vi "Find Average Center.vi"(5 "Position":i32, 6 "Database Entry in":refnum<class "Database Entry.lvclass">, 7 "Tray Number":i32, 8 "Assembly Type":string, 9 "XYZTheta":dbl[](array[numeric]), 10 "Sensor Thickness":dbl, 11 "Gantry In":refnum<k24>) -> (1 "XYZTheta":dbl[](array[numeric]) format="%.6g", 3 "Gantry Out":refnum<k24>, 4 "Database Entry out":refnum<class "Database Entry.lvclass">)   [LabVIEW 2021, in "Component Tray.lvclass"]
uses:
  Component Tray.lvclass
  Find Component.ctl
  Controller/Camera/Machine Vision.ctl
  C:/Program Files (x86)/Aerotech/A3200/LabVIEW/2010/Bin/Aerotech.A3200.dll
  Program Files (x86)/Aerotech/A3200/LabVIEW/2010/Bin/Aerotech.A3200.dll
  Controller/Camera/Camera settings.ctl
  <vilib>/vision/Pattern Matching.llb/IMAQ Pattern Match Advanced Options.ctl
  Assembly/Database Entry/Database Entry.lvclass
  Controller/Camera/Edmund Optics/Edmund Optics.lvclass
  C:/Users/HEP/Documents/GitHub/Gantry/UCSB-Gantry-HEP-main/Classes/Controller/Camera/Camera.lvclass
  <vilib>/picture/picture.llb/Draw 4-Bit Pixmap.vi
  Controller/Camera/Camera.lvclass
  Controller/Motion/A3200/A3200.lvclass
  Controller/Motion/Motion.lvclass
  <vilib>/vision/NI_Vision_Development_Module.lvlib
  <vilib>/vision/Image Controls.llb/IMAQ Image.ctl
  <vilib>/vision/driver/NI_Vision_Acquisition_Software.lvlib
panel:
  out "Sensor ID match DB?":bool
  in  "Algorithm":i32(ring)=2 items=["All", "Low Discrepancy Sampling", "Grayscale Value Pyramid", "Gradients Pyramid"]
  in  "Parameters":T1={"Number of Matches Requested"=1, "Minimum Match Score"=800.0, "Angle Ranges"=[]}
  in  "ROI Descriptor":T2 {"Contours"."Type" items=["No Selection", "Point", "Line", "Rectangle", "Oval", "Polygon", "Freehand Region", "Annulus", "Unused2", "Unused3", "Broken Line", "Freehand Line", "Rotated Rectangle"]}
  in  "Advanced Options":cluster{"Item":T3, "Value":dbl}[](array[cluster]) {"Item" items=["LD Sampling - Minimum Constrast"=0, "LD Sampling - Enable Subpixel Accuracy"=1, "LD Sampling - Search Strategy"=2, "LD Sampling - Subpixel Iterations"=3, "LD Sampling - Subpixel Tolerance"=4, "LD Sampling - Initial Match List Length"=5, "LD Sampling - Match List Reduction Factor"=6, "LD Sampling - Initial Step Size"=7, "LD Sampling - Intermediate Angular Accuracy"=8, "-"=9, "Pyramid - Max Pyramid Level"=100, "Pyramid - Minimum Contrast"=102, "Pyramid - Enable Subpixel Accuracy"=103, "Pyramid - Subpixel Iterations"=104, "Pyramid - Subpixel Tolerance"=105, "Pyramid - Initial Match List Length"=106, "Pyramid - Match List Reduction Factor"=107, "Pyramid - Intermediate Angular Accuracy"=108, "Pyramid - Process Border Matches"=109, "Pyramid - Min Match Separation Distance"=111, "Pyramid - Min Match Separation Angle"=112, "Pyramid - Max Match Overlap"=113, "Pyramid - Max Cache in MB"=114, "Pyramid - Clear Cache"=115, "Pyramid - Enable Accurate Score Computation"=116, "Pyramid - Interpolation Method For Score Computation"=117, "Pyramid - Enable Target To Template Score"=118, "-"=119, "Enable Defect Map"=200]}
  out "Sensor ID digits":i32[](array[numeric])
  out "Checking Sensor ID":bool
  out "All Matches XY":sgl[][](array[numeric])
  out "Match found?":bool
  in  "Focus":bool
  out "Gantry":dbl[](array[numeric]) format="%.6g"
  out "Sum":dbl[](array[numeric]) format="%.6g"
  in  "Machine Vision":T4
  out "Radius (Real-World)":dbl
  out "Standard Variation":sgl
  out "Maximal Value":sgl
  out "Average Strength":dbl
  out "Instructions":string
  out "Camera":dbl[](array[numeric])
  out "Image":T5(plugin-control)
  in  "Enter Manual Mode":bool
  out "Manual Mode On":bool
  in  "Auto Submit":bool
  out "Tray and Position":string
  out "Sensor ID":picture[](array[picture])
  out "Sensor ID":string
  out "predicted fiducials":dbl[][](array[numeric])
  out "Current Z High Speed":dbl
  out "Current XY High Speed":dbl
  out "current Z low speed":dbl
  out "current XY speed":dbl
  in  "Z high":dbl=12.5
  in  "XY high":dbl=50.0
  in  "Z low":dbl=0.05
  in  "XY low":dbl=0.1
  in  "Predict fiducials":bool
  out "Low Speed":bool
  out "X":bool
  out "Y":bool
  out "Z":bool
  out "High Speed":bool
  in  "Go to CH191/FD5":bool
  in  "Go to CH197/FD4":bool
  out "Program Done?":bool
  out "Sensor ID Location":dbl[](array[numeric])
  in  "Go to Sensor ID":bool
  out "CH1 XYZ":dbl[](array[numeric])
  out "CH1 correct?":bool
  in  "Go to CH1":bool
  out "All fiducials recorded":bool
  in  "Override camera presets":bool
  in  "Camera settings":T6={"Gamma"=1.6, "Gain"=0, "Sharpness"=0, "Contrast"=0.0, "Exposure"=0.0078125} {"Exposure" min=0.000244140625 max=0.5 scale=0.0002..0.5; "Contrast" min=0.0 max=1.0 scale=0.001..1.0; "Sharpness" min=0 max=2 step=1 scale=0.0..2.0; "Gain" min=0 max=100 step=1 scale=0.1..100.0; "Gamma" min=0.01 max=10.0 scale=0.01..10.0}
  out "CH197/FD4 XYZ":dbl[](array[numeric]) format="%.6g"
  out "CH8/FD2 XYZ":dbl[](array[numeric]) format="%.6g"
  out "CH191/FD5 XYZ":dbl[](array[numeric]) format="%.6g"
  out "CH1/FD1 XYZ":dbl[](array[numeric]) format="%.6g"
  in  "Record CH8/FD2":bool
  in  "Record CH197/FD4":bool
  in  "Record CH191/FD5":bool
  in  "Record CH1/FD1":bool
  in  "Go to CH8/FD2":bool
  in  "Go to CH1/FD1":bool
  in  "Joystick":bool
  in  "Go to Center":bool
  in  "Component":T7
  in  "Stop Program":bool
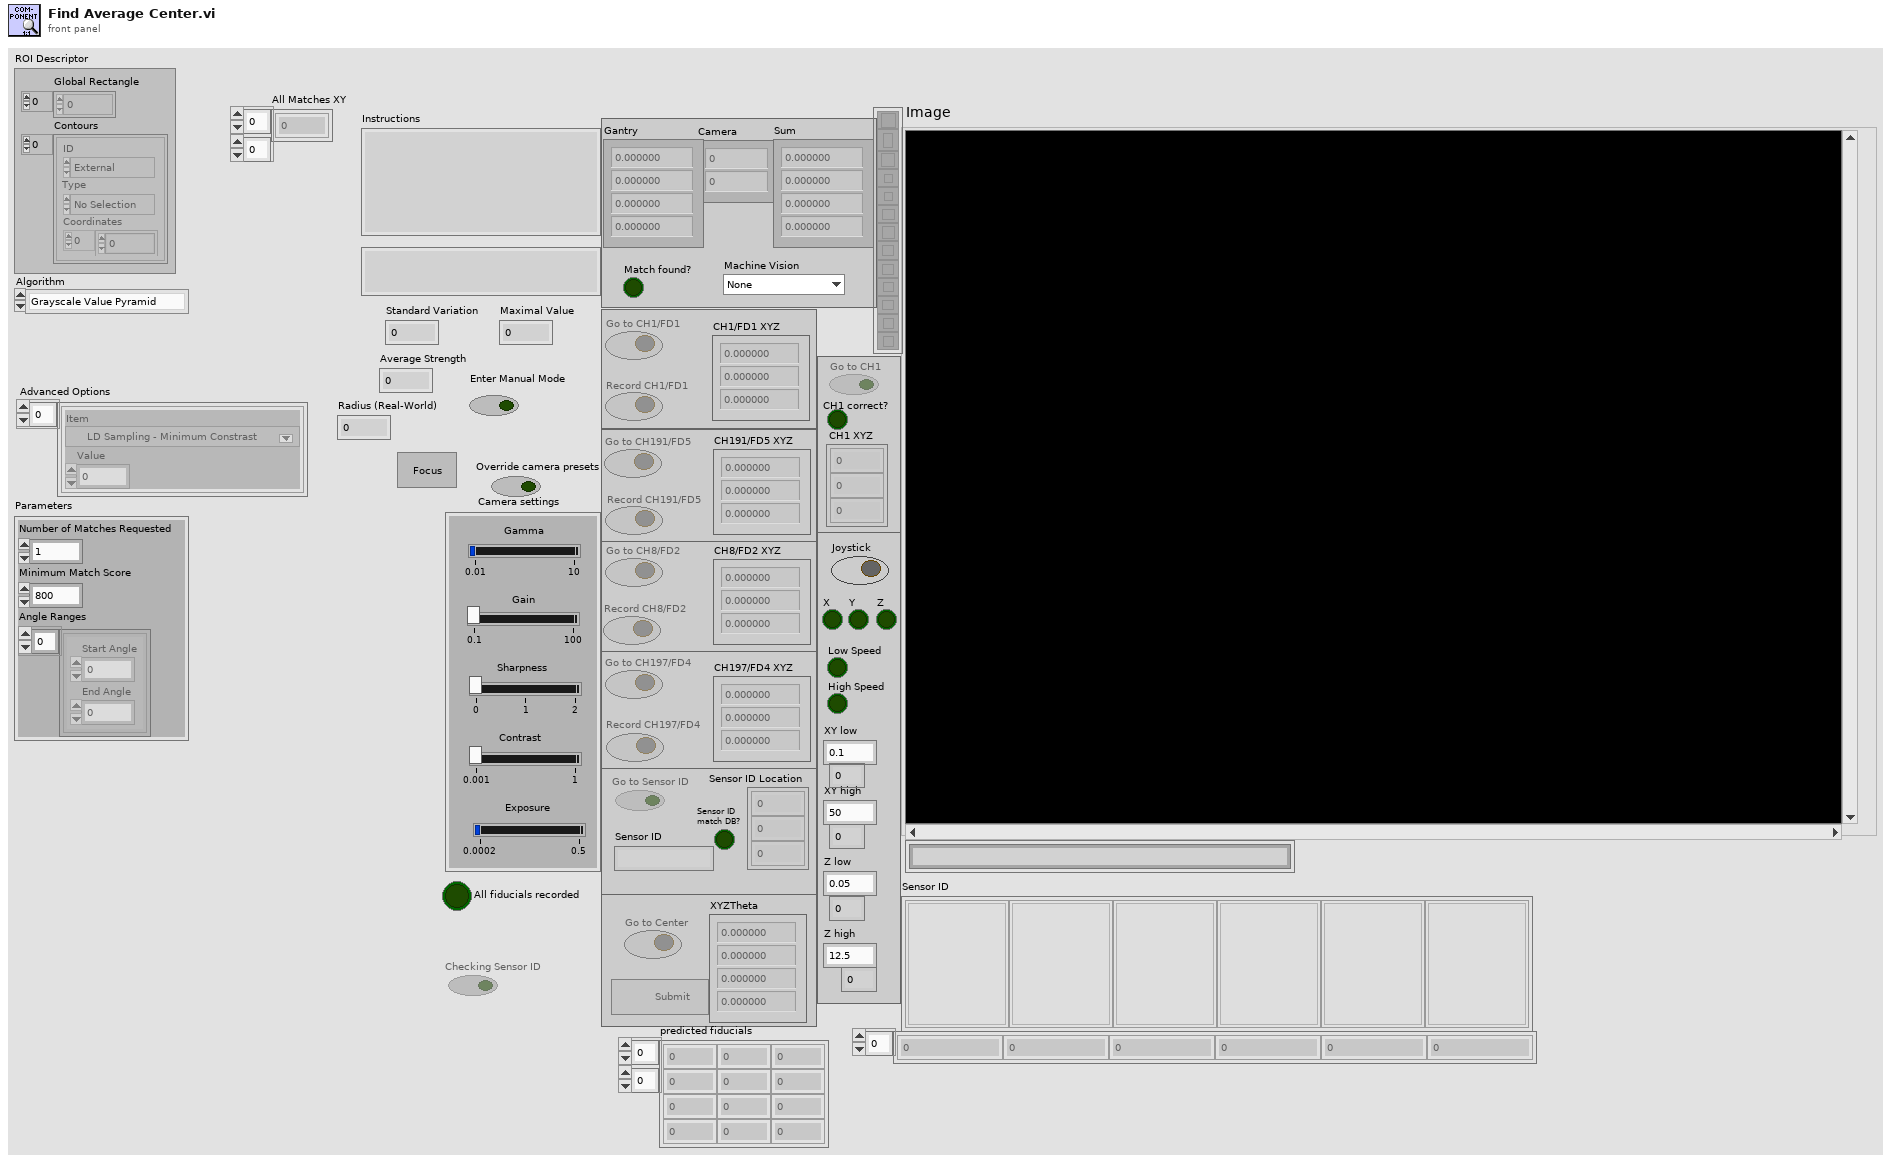
[diagram p1: front panel]
types:
  T1 = cluster{"Number of Matches Requested":i32, "Minimum Match Score":sgl, "Angle Ranges":cluster{"Start Angle":sgl, "End Angle":sgl}[]}
  T2 = typedef "ROI Descriptor" = cluster{"Global Rectangle":i32[], "Contours":cluster{"ID":enum32{"External", "Internal"}, "Type":u32, "Coordinates":i32[]}[]}
  T3 = typedef "IMAQ Pattern Match Advanced Options.ctl" = u16
  T4 = typedef "Camera.lvclass/Machine Vision.ctl" = enum16{"None", "Assembly Tray Circle", "Assembly Tray Fiducial", "Partial Hexaboard", "sensor edge init", "HB edge init", "sensor edge pos1", "sensor edge pos2", "HB edge pos1", "HB edge pos2", "Sensor CH1-2", "HB CH1", "HB CH2", "V3 Sensor Circle", "Hexaboard Circle", "sensor CH1 check", "HB CH1 check ", "sensor ID"}
  T5 = typedef "IMAQ Image.ctl" = refnum<image>
  T6 = typedef "Camera.lvclass/Camera settings.ctl" = cluster{"Gamma":dbl, "Gain":i64, "Sharpness":i64, "Contrast":dbl, "Exposure":dbl}
  T7 = typedef "Component Tray.lvclass/Find Component.ctl" = cluster{"New Fiducials":dbl[], "Past Fiducials":dbl[][], "XYZTheta":dbl[], "Fiducials Path":path, "Position":i32, "CH1 Location":dbl[], "Sensor ID Location":dbl[], "initial rotation":dbl[], "CH2 location":dbl[], "max std variation":dbl, "max strength":dbl, "CH2 pattern matching":T4, "Fiducial Circle":T4, "Get Edge":T4, "Pos multiplier":dbl, "time to wait":u32, "fiducial to edge":dbl, "Protomodule?":bool, "Assembly Type":string, "CH1 to CH2":dbl, "Tray Number":string, "fiducial radius":dbl, "4 fiducials?":bool, "CH1 check":T4, "Edge Scan":T4, "CH1 pattern matching":T4, "Sensor Thickness":dbl, "Previous Avgs":dbl[][], "avg value count":dbl[]}
  T8 = enum8{"Enabled", "Disabled", "Disabled and Grayed Out"}
  T9 = enum16{"None", "Assembly Tray Circle", "Assembly Tray Fiducial", "Partial Hexaboard", "sensor edge init", "HB edge init", "sensor edge pos1", "sensor edge pos2", "HB edge pos1", "HB edge pos2", "Sensor CH1-2", "HB CH1", "HB CH2", "V3 Sensor Circle", "Hexaboard Circle", "sensor CH1 check", "HB CH1 check "}
  T10 = cluster{"Average Strength":dbl, "Radius (Real-World)":dbl, "Match found?":bool, "initial angle":sgl, "Global Report":cluster{"Mean Value":sgl, "Standard Variation":sgl, "Minimal Value":sgl, "Maximal Value":sgl, "Area (calibrated)":sgl, "Area (pixels)":u32, "%":sgl, "Calibration Valid":bool}}
  T11 = typedef "IMAQ GM Match Report.ctl" = cluster{"Position":cluster{"x":sgl, "y":sgl}, "Angle":sgl, "Scale":sgl, "Score":sgl, "Bounding Box":cluster{"x":sgl, "y":sgl}[], "Contrast Reversed":bool, "Occlusion %":sgl, "Template Target Curve Score":sgl, "Target Template Curve Score":sgl, "Correlation Score":sgl}
  T12 = cluster{"Mean Value":sgl, "Standard Variation":sgl, "Minimal Value":sgl, "Maximal Value":sgl, "Area (calibrated)":sgl, "Area (pixels)":u32, "%":sgl, "Calibration Valid":bool}
  T13 = cluster{"left":i16, "top":i16, "right":i16, "bottom":i16}
  T14 = cluster{"Algorithm":i32, "Number of Matches Requested":i32, "Minimum Match Score":sgl, "SubPixel Accuracy":bool, "Rotation Angle Ranges":cluster{"Start":sgl, "End":sgl}[], "Show Search Area":bool, "Show Result":bool}
  T15 = typedef "File Paths.ctl" = cluster{"Glue Pattern Folder":path, "Carrier Tray Folder":path, "Pick Up Tool Fixture Folder":path, "Components Folder":path, "Bellows Tool Offset.txt":path, "Pick Up Tool Offset.txt":path, "Dispense Tip Offset.txt":path, "Log Files":path, "Gantry Assembly Map.txt":path, "Syringe and offset map.txt":path, "Controllers Folder":path, "Local dbase config":path}
  T16 = typedef "imagedata.ctl" = cluster{"image type":i32, "image depth":i32, "image":u8[], "mask":u8[], "colors":u32[], "Rectangle":cluster{"left":i16, "top":i16, "right":i16, "bottom":i16}}
  T17 = cluster{"left":dbl, "top":dbl, "right":dbl, "bottom":dbl}
  T18 = cluster{"Position":cluster{"x":sgl, "y":sgl}, "Angle":sgl, "Scale":sgl, "Score":sgl, "Bounding Box":cluster{"x":sgl, "y":sgl}[]}[]
  T19 = cluster{"[0]":i32, "[1]":i32, "[2]":i32, "[3]":i32, "[4]":i32}
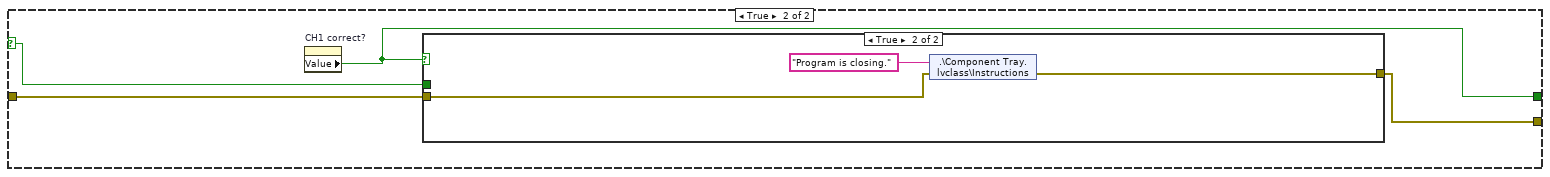
[diagram p6: hidden frame]
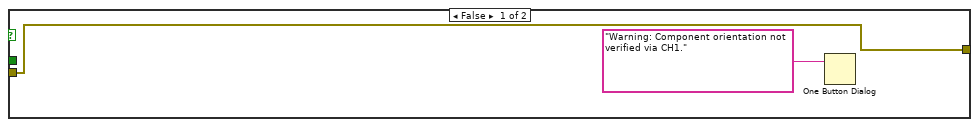
[diagram p7: hidden frame]
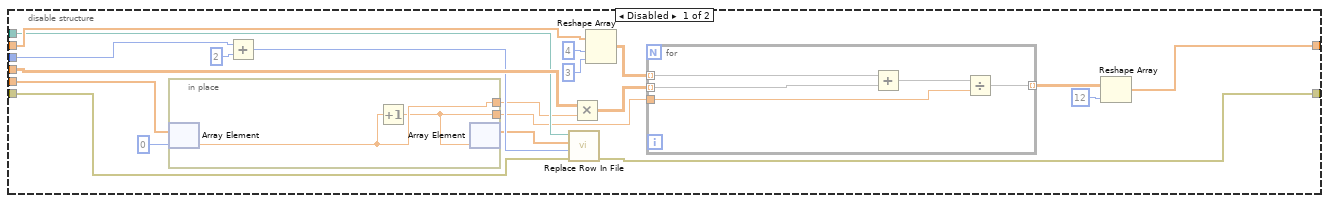
[diagram p9: hidden frame]
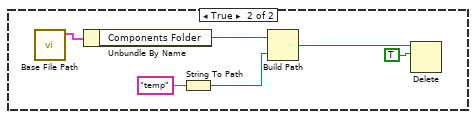
[diagram p10: hidden frame]
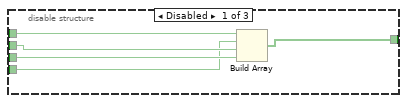
[diagram p12: hidden frame]
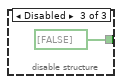
[diagram p13: hidden frame]
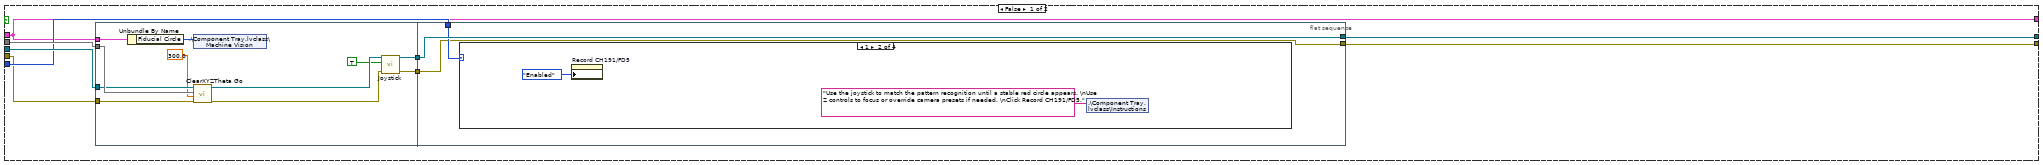
[diagram p14: hidden frame]
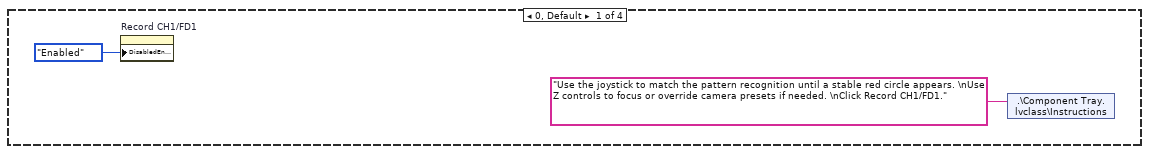
[diagram p15: hidden frame]
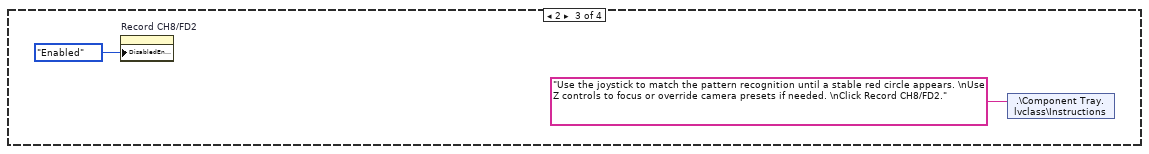
[diagram p16: hidden frame]
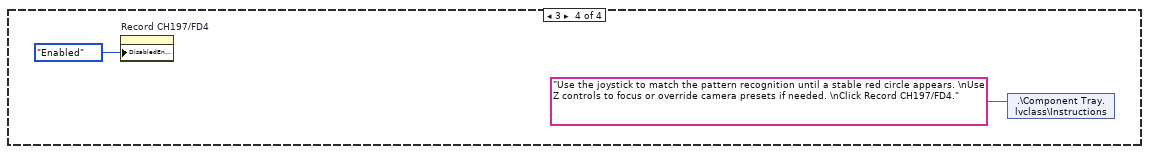
[diagram p17: hidden frame]
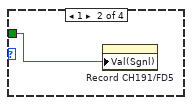
[diagram p18: hidden frame]
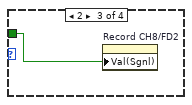
[diagram p19: hidden frame]
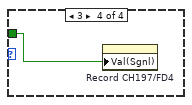
[diagram p20: hidden frame]
diagram:
  n1 = flat-sequence {
    tunnel: [w20] -> w13
    tunnel: [w22] -> w11
    tunnel: ["Gantry In"] -> w9
    tunnel: ["Position"] -> w8
    tunnel: [w28] -> w6
    tunnel: w13 -> [w28]
    tunnel: [w27] -> w5
    tunnel: w11 -> [w27]
    tunnel: [w26] -> w4
    tunnel: w9 -> [w26]
    tunnel: [w25] -> w3
    tunnel: w8 -> [w25]
    tunnel: [w24] -> w1
    tunnel: [w34] -> w12
    tunnel: w6 -> [w34]
    tunnel: w5 -> [w37]
    tunnel: [w37] -> w10
    tunnel: [w36] -> w2
    tunnel: w4 -> [w36]
    tunnel: [w35] -> w7
    tunnel: w3 -> [w35]
    frame #0 {
      w22 = refnum<class "Edmund Optics.lvclass"> refnum  # Edmund Optics.lvclass
      (unwired) 1 ("y")
      n2 = call "Find Average Center Setup.vi"("Sensor Thickness"="Sensor Thickness", "Assembly Type"="Assembly Type", "Position"="Position", "Tray Number"="Tray Number", "XYZTheta"="XYZTheta", "Component"="Component") -> ("output cluster"=w20:T7)  [unwired: 5 in]
    }
    frame #1 {
      n3 = control-ref of="This VI"() -> (w29:refnum<vi>)
      n4 = invoke class="VI" method="Default Vals.Reinit All"(reference=w29) -> (error out=w24:errorcluster)  [unwired: 2 in, 2 out]
    }
    frame #2 {
      n5 = Unbundle By Name(w34) -> ("4 fiducials?"=w30:bool)
      n6 = Select(t=T8."Enabled" ("Disabled"), s=w30, f=T8."Disabled and Grayed Out" ("Disabled")) -> (s? t:f=w31:T8)
      n7 = property on="CH197/FD4 XYZ" class="Arr (strict)"("DisabledEnum"=w31) -> ()  [unwired: 2 in, 2 out]
      n8 = property on="Record CH191/FD5" class="Bool (strict)"("DisabledEnum"=w31) -> ()  [unwired: 2 in, 2 out]
      n9 = property on="CH191/FD5 XYZ" class="Arr (strict)"("DisabledEnum"=w31) -> ()  [unwired: 2 in, 2 out]
      n10 = property on="Go to CH191/FD5" class="Bool (strict)"("DisabledEnum"=w31) -> ()  [unwired: 2 in, 2 out]
      n11 = property on="Predict fiducials" class="Bool (strict)"("DisabledEnum"=w31) -> ()  [unwired: 2 in, 2 out]
      n12 = property on="Record CH197/FD4" class="Bool (strict)"("DisabledEnum"=w31) -> ()  [unwired: 2 in, 2 out]
      n13 = property on="Go to CH197/FD4" class="Bool (strict)"("DisabledEnum"=w31) -> ()  [unwired: 2 in, 2 out]
    }
  }
  n14 = while {
    shift-right: [w62] -> _
    shift-left: w10 -> [w64]
    shift-right: [w45] -> _
    shift-left: w2 -> [w47]
    i -> [w59]
    stop <- w43 stop-if-true
    n15 = in-place {
      in-place-border: [w90] -> w46
      in-place-border: w47 -> [w72]
      # "Joystck Status"
      n16 = call "Get Joytick Status.vi"("Gantry In"=w72) -> ("JoystickLowSpeedActive"=w94:bool, "Joystick Status"=w95:bool[], "Gantry Out"=w91:refnum<k24>, "High Speeds"=w79:dbl[], "Low Speeds"=w78:dbl[])  [unwired: 5 in, 1 out]
      n17 = Build Array("XY low", "XY low", "XY low", "Z low") -> (w85:dbl[])
      n18 = Build Array("XY high", "XY high", "XY high", "Z high") -> (w84:dbl[])
      n19 = call "Set Joystick Speed.vi"("High Speed Inputs"=w84, "Low Speed Inputs"=w85, "Gantry"=w91) -> ("Controller Out"=w90:refnum<k24>)  [unwired: 7 in, 1 out]
      n20 = Or Array Elements(Boolean array=w95) -> (logical OR=w92:bool)
      n21 = Not(x=w94) -> (.not. x?=w93:bool)
      n22 = Index Array(array=w79) -> (element #1=→"Current XY High Speed":dbl, element #3=→"Current Z High Speed":dbl)  [unwired: 3 in, 1 out]
      n23 = Index Array(array=w78) -> (element #1=→"current XY speed":dbl, element #3=→"current Z low speed":dbl)  [unwired: 3 in, 1 out]
      n24 = Index Array(array=w95) -> (element #1=→"X":bool, element #2=→"Y":bool, element #3=→"Z":bool)  [unwired: 3 in]
      n25 = And(x=w93, y=w92) -> (x .and. y?=→"High Speed":bool)
      n26 = And(x=w92, y=w94) -> (x .and. y?=→"Low Speed":bool)
    }
    n27 = local read "Checking Sensor ID"() -> (w38:bool)
    n28 = shared-variable ".\\Component Tray.lvclass\\Instructions"() -> (→"Instructions":string)  [unwired: 1 in, 1 out]
    n29 = property on="Manual Mode On" class="Bool (strict)"() -> ("Value"=w40:bool)  [unwired: 2 in, 2 out]
    n30 = shared-variable ".\\Component Tray.lvclass\\Manual Mode"("Enter Manual Mode") -> ()  [unwired: 1 in, 1 out]
    n31 = Or(x=w40, y=w38) -> (x .or. y?=w39:bool)
    n32 = case shown="True" w39 {
      tunnel: [w96 "Machine Vision"] -> w48
      frame False {
        n33 = shared-variable ".\\Component Tray.lvclass\\Machine Vision"() -> (w96:T9)  [unwired: 1 in, 1 out]
      }
      frame True {
      }
    }
    n34 = local read "Program Done?"() -> (w43:bool)
    n35 = Equal To 0?(x=w59) -> (x = 0?=w58:bool)
    n36 = call "Camera.vi"("Camera in"=w64, "Stop"=w43, "Machine Vision"=w48, "Camera settings"="Camera settings", "Loop 0"=w58, "Override presets"="Override camera presets") -> ("All Matches XY"=→"All Matches XY":sgl[][], "Camera out"=w62:refnum<class "Edmund Optics.lvclass">, "output cluster"=w57:T10, "pattern matching"=w50:T11, "Image"=→"Image":T5, "Camera"=w42:dbl[])  [unwired: 6 in, 2 out]
    "Camera" <- w42
    n37 = Unbundle By Name(w57) -> ("Average Strength"=w56:dbl, "Radius (Real-World)"=w55:dbl, "Match found?"=w54:bool, "Global Report"=w53:T12)
    "Average Strength" <- w56
    "Radius (Real-World)" <- w55
    "Match found?" <- w54
    n38 = shared-variable ".\\Component Tray.lvclass\\pattern matching"(w50) -> ()  [unwired: 1 in, 1 out]
    n39 = shared-variable ".\\Component Tray.lvclass\\Camera"(w42) -> ()  [unwired: 1 in, 1 out]
    n40 = in-place {
      in-place-border: w46 -> [w67]
      in-place-border: [w66] -> w45
      in-place-border: w42 -> [w65]
      # "Current Position"
      n41 = call "Get Current Position.vi"("Gantry In"=w67) -> ("XYZTheta Out"=w70:dbl[], "Gantry Out"=w66:refnum<k24>)  [unwired: 8 in, 1 out]
      "Gantry" <- w70
      n42 = Reshape Array(w65, 4 ("dimension size")) -> (w69:dbl[])
      n43 = Add(x=w70, y=w69) -> (x+y=→"Sum":dbl[])
    }
    n44 = shared-variable ".\\Component Tray.lvclass\\Average Strength"(w56) -> ()  [unwired: 1 in, 1 out]
    n45 = shared-variable ".\\Component Tray.lvclass\\Radius (Real-World)"(w55) -> ()  [unwired: 1 in, 1 out]
    n46 = shared-variable ".\\Component Tray.lvclass\\Match found?"(w54) -> ()  [unwired: 1 in, 1 out]
    n47 = Unbundle By Name(w53) -> ("Standard Variation"=w52:sgl, "Maximal Value"=w51:sgl)
    "Maximal Value" <- w51
    "Standard Variation" <- w52
    n48 = shared-variable ".\\Component Tray.lvclass\\Standard Variation"(w52) -> ()  [unwired: 1 in, 1 out]
    n49 = shared-variable ".\\Component Tray.lvclass\\Maximal Value"(w51) -> ()  [unwired: 1 in, 1 out]
  }
  n50 = while {
    shift-right: [w107] -> _
    shift-left: w12 -> [w100]
    shift-right: [w105] -> w14
    shift-left: w2 -> [w106]
    tunnel: w7 -> [w101]
    shift-right: [w98] -> _
    shift-left: w1 -> [w99]
    i -> [w104]
    stop <- w108 stop-if-true
    n51 = event shown="[10] \"Go to Sensor ID\": Value Change" {
      selector: _ -> [_ _ _ _ _ _ _ _ _ _ _]
      dyn-events: _ -> [_ _ _ _ _ _ _ _ _ _ _]
      timeout: _ -> [_ _ _ _ _ _ _ _ _ _ _]
      tunnel: [_ _ w147 _ _ _ _ _ _ _ _] -> w108
      tunnel: w100 -> [w126 w127 w151 w233 w385 w465 w492 w500 w542 w689 w697]
      tunnel: [w126 w127 w151 w229 w392 w464 w492 w500 w542 w689 w697] -> w107
      tunnel: w106 -> [w125 w134 w152 w237 w408 w469 w491 w499 w548 w691 w709]
      tunnel: [w125 w131 w150 w231 w386 w469 w489 w497 w546 w691 w708] -> w105
      tunnel: w99 -> [w124 w138 w144 w223 w391 w462 w488 w495 w538 w686 w706]
      tunnel: [w124 w128 w145 w221 w389 w462 w487 w493 w536 w686 w705] -> w98
      event Timeout {
        n52 = event-data() -> ()  [unwired: 1 in, 3 out]
      }
      event "Focus": Value Change {
        n53 = event-data() -> ()  [unwired: 1 in, 6 out]
        n54 = Unbundle By Name(w127) -> ()  [unwired: 1 out]
        n55 = shared-variable ".\\Component Tray.lvclass\\Instructions"(error in=w138) -> (w140:string, error out=w136:errorcluster)
        n56 = call "Joystick.vi"("error in (no error)"=w136, "Joystick"=FALSE, "Gantry In"=w134) -> ("error out"=w135:errorcluster, "Gantry Out"=w133:refnum<k24>)  [unwired: 7 in]
        n57 = shared-variable ".\\Component Tray.lvclass\\Instructions"("Finding best focus. Wait for movement to stop." ("Instructions"), error in=w135) -> (error out=w142:errorcluster)
        n58 = call "Best Focus.vi"("Component"=w127, "error in (no error)"=w142, "Inc by"=0.02, "Gantry In"=w133) -> ("error out"=w141:errorcluster, "Gantry Out"=w130:refnum<k24>)  [unwired: 4 in, 2 out]
        n59 = shared-variable ".\\Component Tray.lvclass\\Instructions"(w140, error in=w141) -> (error out=w129:errorcluster)
        n60 = call "Joystick.vi"("error in (no error)"=w129, "Joystick"=TRUE, "Gantry In"=w130) -> ("error out"=w128:errorcluster, "Gantry Out"=w131:refnum<k24>)  [unwired: 7 in]
      }
      event "Stop Program", "Auto Submit": Value Change {
        n61 = event-data() -> ()  [unwired: 1 in, 6 out]
        n62 = flat-sequence {
          frame #0 {
          }
          frame #1 {
            n63 = property on="Auto Submit" class="Bool (strict)"("Value"=FALSE ("Auto Submit")) -> ()  [unwired: 2 in, 2 out]
          }
        }
        n64 = property on="All fiducials recorded" class="Bool (strict)"() -> ("Value"=w149:bool)  [unwired: 2 in, 2 out]
        n65 = case shown="False" w149 {
          selector: w149 -> [w154 w159]
          tunnel: [w154 w158] -> w148
          tunnel: [w153 w157] -> w146
          tunnel: w144 -> [w153 w156]
          frame False {
            n66 = One Button Dialog(message="Warning: At least one fiducial not recorded.") -> ()  [unwired: 1 in, 1 out]
          }
          frame True {
            n67 = property on="CH1 correct?" class="Bool (strict)"() -> ("Value"=w158:bool)  [unwired: 2 in, 2 out]
            n68 = case shown="True" w158 {
              tunnel: w159 -> [_ _]
              tunnel: w156 -> [w160 w163]
              tunnel: [w160 w162] -> w157
              frame False {
                n69 = One Button Dialog(message="Warning: Component orientation not verified via CH1.") -> ()  [unwired: 1 in, 1 out]
              }
              frame True {
                n70 = shared-variable ".\\Component Tray.lvclass\\Instructions"("Program is closing." ("Instructions"), error in=w163) -> (error out=w162:errorcluster)
              }
            }
          }
        }
        n71 = case shown="True" w148 {
          selector: w148 -> [w167 w185]
          tunnel: w152 -> [w168 w184]
          tunnel: w151 -> [_ w182]
          tunnel: [w168 w183] -> w150
          tunnel: [w167 w185] -> w147
          tunnel: w146 -> [w166 w173]
          tunnel: [w166 w170] -> w145
          frame False {
          }
          frame True {
            n72 = Unbundle By Name(w182) -> ("Fiducials Path"=w175:path, "New Fiducials"=w177:dbl[], "Position"=w174:i32, "Protomodule?"=w181:bool, "Previous Avgs"=w178:dbl[][], "avg value count"=w169:dbl[])
            n73 = call "Joystick.vi"("error in (no error)"=w173, "Joystick"=FALSE, "Gantry In"=w184) -> ("error out"=w172:errorcluster, "Gantry Out"=w183:refnum<k24>)  [unwired: 7 in]
            n74 = case shown="False" w181 {
              frame False {
              }
              frame True {
                n75 = call "Base File Path.vi"() -> ("Paths Out"=w219:T15)  [unwired: 11 in]
                n76 = Unbundle By Name(w219) -> ("Components Folder"=w217:path)
                n77 = String To Path(string="temp") -> (path=w218:path)
                n78 = Build Path(base path=w217, name or relative path=w218) -> (appended path=w220:path)
                n79 = Delete(path (use dialog)=w220, entire hierarchy (F)=TRUE) -> ()  [unwired: 3 in, 3 out]
              }
            }
            n80 = disable-structure shown="Enabled" {
              disable-tunnel: w178 -> [w205 _]
              disable-tunnel: w177 -> [w198 w214]
              disable-tunnel: [w197 w214] -> w176
              disable-tunnel: w175 -> [w196 _]
              disable-tunnel: w174 -> [w195 _]
              disable-tunnel: w172 -> [w192 w213]
              disable-tunnel: [w191 w213] -> w171
              disable-tunnel: w169 -> [w190 _]
              frame Disabled {
                n81 = in-place {
                  in-place-border: [w207] -> w188
                  in-place-border: [w206] -> w187
                  n82 = in-place-array #1(w190, 0) -> (w207:dbl)
                  n83 = Increment(x=w207) -> (x+1=w206:dbl)
                  n84 = in-place-array #1(w206) -> (w189:dbl[])  [unwired: 1 out]
                }
                n85 = Add(x=w195, y=2) -> (x+y=w193:i32)
                n86 = call "Replace Row In File.vi"("error in"=w192, "Index"=w193, "Insert Array"=w189, "Path"=w196) -> ("error out"=w191:errorcluster)  [unwired: 7 in]
                n87 = Multiply(x=w205, y=w188) -> (x*y=w201:dbl[][])
                n88 = Reshape Array(w198, 4 ("dimension size"), 3 ("dimension size")) -> (w202:dbl[][])
                n89 = for {
                  tunnel: w202 -> [w212] mode=indexing
                  tunnel: w201 -> [w211] mode=indexing
                  tunnel: w187 -> [w209]
                  tunnel: [w208] -> w200 mode=indexing
                  n90 = Add(x=w212, y=w211) -> (x+y=w210:dbl[])
                  n91 = Divide(x=w210, y=w209) -> (x/y=w208:dbl[])
                }
                n92 = Reshape Array(w200, 12 ("dimension size")) -> (w197:dbl[])
              }
              frame Enabled {
              }
            }
            n93 = shared-variable ".\\Component Tray.lvclass\\Instructions"("Program is done." ("Instructions")) -> ()  [unwired: 1 in, 1 out]
            n94 = call "Replace Row In File.vi"("error in"=w171, "Index"=w174, "Insert Array"=w176, "Path"=w175) -> ("error out"=w170:errorcluster)  [unwired: 7 in]
          }
        }
        "Program Done?" <- w147
      }
      event "Go to CH1/FD1", "Go to CH8/FD2", "Go to CH197/FD4", "Go to CH191/FD5": Value Change {
        n95 = event-data() -> ()  [unwired: 1 in, 6 out]
        n96 = flat-sequence {
          tunnel: w237 -> [w239]
          tunnel: w233 -> [w238]
          tunnel: [w240] -> w226
          tunnel: [w239] -> w225
          tunnel: [w238] -> w224
          tunnel: [w259] -> w236
          tunnel: [w257] -> w234
          tunnel: [w260] -> w235
          tunnel: [w255] -> w232
          tunnel: [w249] -> w230
          tunnel: [w254] -> w228
          tunnel: [w252] -> w227
          tunnel: w226 -> [w251]
          tunnel: w225 -> [w250]
          tunnel: w224 -> [w249]
          tunnel: w223 -> [w248]
          tunnel: [w246] -> w222
          tunnel: w236 -> [w282]
          tunnel: w235 -> [w281]
          tunnel: w234 -> [w276]
          tunnel: w232 -> [w280]
          tunnel: [w275] -> w231
          tunnel: w230 -> [w274]
          tunnel: [w273] -> w229
          tunnel: w228 -> [w271]
          tunnel: w227 -> [w269]
          tunnel: w222 -> [w265]
          tunnel: [w263] -> w221
          frame #0 {
            n97 = Build Array "Build Array"("Go to CH1/FD1", "Go to CH191/FD5", "Go to CH8/FD2", "Go to CH197/FD4") -> (w240:bool[])
          }
          frame #1 {
            w245 = FALSE ("Go to Top Right Fiducial")
            n98 = property on="Go to CH1/FD1" class="Bool (strict)"("Value"=w245) -> ()  [unwired: 2 in, 2 out]
            n99 = property on="Go to CH191/FD5" class="Bool (strict)"("Value"=w245) -> ()  [unwired: 2 in, 2 out]
            n100 = property on="Go to CH8/FD2" class="Bool (strict)"("Value"=w245) -> ()  [unwired: 2 in, 2 out]
            n101 = property on="Go to CH197/FD4" class="Bool (strict)"("Value"=w245) -> ()  [unwired: 2 in, 2 out]
          }
          frame #2 {
            w262 = T8."Disabled and Grayed Out" ("Disabled")
            n102 = property on="Go to CH1/FD1" class="Bool (strict)"("DisabledEnum"=w262) -> ()  [unwired: 2 in, 2 out]
            n103 = property on="Go to CH1" class="Bool (strict)"("DisabledEnum"=w262) -> ()  [unwired: 2 in, 2 out]
            n104 = property on="Record CH1/FD1" class="Bool (strict)"("DisabledEnum"=w262) -> ()  [unwired: 2 in, 2 out]
            n105 = property on="Go to Center" class="Bool"("DisabledEnum"=w262) -> ()  [unwired: 2 in, 2 out]
            n106 = property on="Record CH191/FD5" class="Bool (strict)"("DisabledEnum"=w262) -> ()  [unwired: 2 in, 2 out]
            n107 = property on="Stop Program" class="Bool"("DisabledEnum"=w262) -> ()  [unwired: 2 in, 2 out]
            n108 = property on="Record CH197/FD4" class="Bool (strict)"("DisabledEnum"=w262) -> ()  [unwired: 2 in, 2 out]
            n109 = property on="Go to CH8/FD2" class="Bool (strict)"("DisabledEnum"=w262) -> ()  [unwired: 2 in, 2 out]
            n110 = property on="Record CH8/FD2" class="Bool (strict)"("DisabledEnum"=w262) -> ()  [unwired: 2 in, 2 out]
            n111 = property on="Go to Sensor ID" class="Bool (strict)"("DisabledEnum"=w262) -> ()  [unwired: 2 in, 2 out]
            n112 = property on="Go to CH191/FD5" class="Bool (strict)"("DisabledEnum"=w262) -> ()  [unwired: 2 in, 2 out]
            n113 = property on="Go to CH197/FD4" class="Bool (strict)"("DisabledEnum"=w262) -> ()  [unwired: 2 in, 2 out]
            n114 = shared-variable ".\\Component Tray.lvclass\\Instructions"("Wait for movement to stop." ("Value (Signaling)"), error in=w248) -> (error out=w247:errorcluster)
            n115 = Unbundle By Name(w249) -> ("Past Fiducials"=w256:dbl[][], "Assembly Type"=w255:string, "4 fiducials?"=w254:bool, "Protomodule?"=w252:bool)
            n116 = Search 1D Array(1D array=w251, element=TRUE) -> (index of element=w257:i32)  [unwired: 1 in]
            n117 = call "Joystick.vi"("error in (no error)"=w247, "Joystick"=FALSE, "Gantry In"=w250) -> ("error out"=w246:errorcluster, "Gantry Out"=w260:refnum<k24>)  [unwired: 7 in]
            n118 = Index Array(array=w256, index (row)=w257) -> (element=w259:dbl[])  [unwired: 1 in]
          }
          frame #3 {
            n119 = Search and Replace String(case sensitive?=TRUE ("ignore case? (F)"), input string=w280, search string="Full", error in=w265) -> (number of replacements=w277:i32, error out=w264:errorcluster)  [unwired: 4 in, 2 out]
            n120 = local read "Manual Mode On"() -> (w268:bool)
            n121 = Not(x=w268) -> (.not. x?=w267:bool)
            n122 = Greater Than 0?(x=w277) -> (x > 0?=w266:bool)
            n123 = disable-structure shown="Enabled" {
              disable-tunnel: [w287 w290 bool[] [FALSE]] -> w272
              disable-tunnel: w271 -> [w286 w289 _]
              disable-tunnel: w269 -> [w285 _ _]
              disable-tunnel: w267 -> [w284 w291 _]
              disable-tunnel: w266 -> [w283 w288 _]
              frame Disabled {
                n124 = Build Array(w284, w283, w286, w285) -> (w287:bool[])
              }
              frame Enabled {
                n125 = Build Array(w291, w289, w288) -> (w290:bool[])
              }
              frame Disabled {
              }
            }
            n126 = And Array Elements(Boolean array=w272) -> (logical AND=w270:bool)
            n127 = case shown="True" w270 {
              tunnel: w282 -> [w301 w332]
              tunnel: w281 -> [w300 w334]
              tunnel: [w299 w328] -> w275
              tunnel: w276 -> [w296 w327]
              tunnel: w274 -> [w295 w333]
              tunnel: [w295 w331] -> w273
              tunnel: w264 -> [w294 w326]
              tunnel: [w293 w324] -> w263
              frame False {
                n128 = flat-sequence {
                  tunnel: w301 -> [w312]
                  tunnel: w300 -> [w311]
                  tunnel: [w309] -> w298
                  tunnel: [w306] -> w297
                  tunnel: w295 -> [w305]
                  tunnel: w294 -> [w302]
                  tunnel: w298 -> [w315]
                  tunnel: w297 -> [w313]
                  tunnel: w296 -> [w314]
                  tunnel: [w315] -> w299
                  tunnel: [w313] -> w293
                  frame #0 {
                    n129 = Unbundle By Name(w305) -> ("Fiducial Circle"=w304:T4)
                    n130 = shared-variable ".\\Component Tray.lvclass\\Machine Vision"(w304) -> ()  [unwired: 1 in, 1 out]
                    n131 = call "ClearXYZTheta Go.vi"("error in (no error)"=w302, "Speed"=300.0, "XYZTheta In"=w312, "Gantry In"=w311) -> ("error out"=w307:errorcluster, "Gantry Out"=w310:refnum<k24>)  [unwired: 5 in, 1 out]
                    n132 = call "Joystick.vi"("error in (no error)"=w307, "Joystick"=TRUE, "Gantry In"=w310) -> ("error out"=w306:errorcluster, "Gantry Out"=w309:refnum<k24>)  [unwired: 7 in]
                  }
                  frame #1 {
                    n133 = case shown="1" w314 {
                      frame 0, Default {
                        n134 = property on="Record CH1/FD1" class="Bool (strict)"("DisabledEnum"=T8."Enabled" ("Disabled")) -> ()  [unwired: 2 in, 2 out]
                        n135 = shared-variable ".\\Component Tray.lvclass\\Instructions"("Use the joystick to match the pattern recognition until a stable red circle appears. \nUse Z controls to focus or override camera presets if needed. \nClick Record CH1/FD1.") -> ()  [unwired: 1 in, 1 out]
                      }
                      frame 1 {
                        n136 = property on="Record CH191/FD5" class="Bool (strict)"("DisabledEnum"=T8."Enabled" ("Disabled")) -> ()  [unwired: 2 in, 2 out]
                        n137 = shared-variable ".\\Component Tray.lvclass\\Instructions"("Use the joystick to match the pattern recognition until a stable red circle appears. \nUse Z controls to focus or override camera presets if needed. \nClick Record CH191/FD5.") -> ()  [unwired: 1 in, 1 out]
                      }
                      frame 2 {
                        n138 = property on="Record CH8/FD2" class="Bool (strict)"("DisabledEnum"=T8."Enabled" ("Disabled")) -> ()  [unwired: 2 in, 2 out]
                        n139 = shared-variable ".\\Component Tray.lvclass\\Instructions"("Use the joystick to match the pattern recognition until a stable red circle appears. \nUse Z controls to focus or override camera presets if needed. \nClick Record CH8/FD2.") -> ()  [unwired: 1 in, 1 out]
                      }
                      frame 3 {
                        n140 = property on="Record CH197/FD4" class="Bool (strict)"("DisabledEnum"=T8."Enabled" ("Disabled")) -> ()  [unwired: 2 in, 2 out]
                        n141 = shared-variable ".\\Component Tray.lvclass\\Instructions"("Use the joystick to match the pattern recognition until a stable red circle appears. \nUse Z controls to focus or override camera presets if needed. \nClick Record CH197/FD4.") -> ()  [unwired: 1 in, 1 out]
                      }
                    }
                  }
                }
              }
              frame True {
                n142 = call "Autolocate Fiducials.vi"("FD Index"=w327, "error in"=w326, "Past Fiducials"=w332, "Component"=w333, "Gantry In"=w334) -> ("error out"=w325:errorcluster, "Wrong Orientation?"=w330:bool, "Component Out"=w331:T7, "Gantry Out"=w329:refnum<k24>)  [unwired: 3 in]
                n143 = case shown="False" w330 {
                  tunnel: w329 -> [w338 w347]
                  tunnel: [w338 w346] -> w328
                  tunnel: w327 -> [w337 _]
                  tunnel: w325 -> [w335 w348]
                  tunnel: [w335 w343] -> w324
                  frame False {
                    n144 = case shown="0, Default" w337 {
                      tunnel: TRUE ("Value (Signaling)") -> [w339 w340 w341 w342]
                      frame 0, Default {
                        n145 = property on="Record CH1/FD1" class="Bool (strict)"("Val(Sgnl)"=w339) -> ()  [unwired: 2 in, 2 out]
                      }
                      frame 1 {
                        n146 = property on="Record CH191/FD5" class="Bool (strict)"("Val(Sgnl)"=w340) -> ()  [unwired: 2 in, 2 out]
                      }
                      frame 2 {
                        n147 = property on="Record CH8/FD2" class="Bool (strict)"("Val(Sgnl)"=w341) -> ()  [unwired: 2 in, 2 out]
                      }
                      frame 3 {
                        n148 = property on="Record CH197/FD4" class="Bool (strict)"("Val(Sgnl)"=w342) -> ()  [unwired: 2 in, 2 out]
                      }
                    }
                  }
                  frame True {
                    n149 = flat-sequence {
                      tunnel: w348 -> [w352]
                      tunnel: w347 -> [w351]
                      tunnel: [w350] -> w345
                      tunnel: [w349] -> w344
                      tunnel: [w376] -> w346
                      tunnel: w345 -> [w376]
                      tunnel: w344 -> [w370]
                      tunnel: [w369] -> w343
                      frame #0 {
                        n150 = Two Button Dialog(message="Warning: Automatic fiducial location failed.\nVerify that CH1 is aligned with the etching on the tray.", 1:"Reposition component" ("F button name (\"Cancel\")"), 2:"CH1 is correct" ("T button name (\"OK\")")) -> (T button?=w353:bool)
                        n151 = case shown="True" w353 {
                          tunnel: w352 -> [w363 w368]
                          tunnel: w351 -> [w360 w367]
                          tunnel: [w359 w367] -> w350
                          tunnel: [w357 w368] -> w349
                          frame False {
                            n152 = call "ClearXYZTheta Go.vi"("error in (no error)"=w363, "Speed"=300.0, "XYZTheta In"=dbl[] [650.0, 650.0, 5.0, 0.0], "Gantry In"=w360) -> ("error out"=w358:errorcluster, "Gantry Out"=w359:refnum<k24>)  [unwired: 5 in, 1 out]
                            n153 = while {
                              shift-right: [w365] -> w357
                              shift-left: w358 -> [w366]
                              stop <- w364 stop-if-true
                              n154 = call "Prompt User for Input"("error in (no error)"=w366) -> ("CH1 correct?"=w364:bool, "error out"=w365:errorcluster)  [unwired: 16 in, 1 out]
                            }
                          }
                          frame True {
                          }
                        }
                      }
                      frame #1 {
                        n155 = Two Button Dialog(message="Restart automatic fiducial location or manually find fiducials?", 1:"Enter manual mode" ("F button name (\"Cancel\")"), 2:"Restart automatic mode" ("T button name (\"OK\")")) -> (T button?=w372:bool)
                        n156 = case shown="True" w372 {
                          tunnel: TRUE ("Value (Signaling)") -> [w379 w382]
                          tunnel: w370 -> [w378 w381]
                          tunnel: [w377 w380] -> w369
                          frame False {
                            n157 = property on="Enter Manual Mode" class="Bool (strict)"(error in=w378, "Val(Sgnl)"=w379) -> (error out=w377:errorcluster)  [unwired: 1 in, 1 out]
                          }
                          frame True {
                            n158 = property on="Go to CH1/FD1" class="Bool (strict)"(error in=w381, "Val(Sgnl)"=w382) -> (error out=w380:errorcluster)  [unwired: 1 in, 1 out]
                          }
                        }
                      }
                    }
                  }
                }
              }
            }
          }
        }
      }
      event "Record CH1/FD1", "Record CH191/FD5", "Record CH197/FD4", "Record CH8/FD2": Value Change {
        n159 = event-data() -> ()  [unwired: 1 in, 1 out]
        n160 = call "Get Current Position.vi"("error in (no error)"=w391, "Gantry In"=w408) -> ("error out"=w384:errorcluster, "XYZTheta Out"=w388:dbl[], "Gantry Out"=w387:refnum<k24>)  [unwired: 7 in]
        n161 = flat-sequence {
          tunnel: ["Record CH1/FD1"] -> _
          tunnel: [w431] -> w396
          frame #0 {
            n162 = Build Array "Build Array"("Record CH1/FD1", "Record CH191/FD5", "Record CH8/FD2", "Record CH197/FD4") -> (w431:bool[])
          }
          frame #1 {
            w436 = FALSE ("Record CH1/FD1")
            n163 = property on="Record CH1/FD1" class="Bool (strict)"("Value"=w436) -> ()  [unwired: 2 in, 2 out]
            n164 = property on="Record CH191/FD5" class="Bool (strict)"("Value"=w436) -> ()  [unwired: 2 in, 2 out]
            n165 = property on="Record CH197/FD4" class="Bool (strict)"("Value"=w436) -> ()  [unwired: 2 in, 2 out]
            n166 = property on="Record CH8/FD2" class="Bool (strict)"("Value"=w436) -> ()  [unwired: 2 in, 2 out]
          }
        }
        n167 = disable-structure shown="Enabled" {
          disable-tunnel: w388 -> [w420 _]
          disable-tunnel: w387 -> [w415 w430]
          disable-tunnel: [w414 w430] -> w386
          disable-tunnel: w385 -> [w413 _]
          disable-tunnel: w384 -> [w412 w429]
          disable-tunnel: [w411 w429] -> w383
          frame Disabled {
            n168 = Index Array(array=w420, index=2) -> (element=w418:dbl)
            n169 = Less?(x=w418, y=50.0) -> (x < y?=w416:bool)
            n170 = case shown="True" w416 {
              tunnel: w415 -> [w422 w428]
              tunnel: [w422 w427] -> w414
              tunnel: w413 -> [_ w426]
              tunnel: w412 -> [w421 w425]
              tunnel: [w421 w424] -> w411
              frame False {
              }
              frame True {
                n171 = call "Temp Joystick.vi"("error in (no error)"=w425, "Fiducial?"=TRUE ("Dialog?"), "Component"=w426, "Gantry In"=w428) -> ("error out"=w424:errorcluster, "Gantry Out"=w427:refnum<k24>)  [unwired: 5 in, 1 out]
              }
            }
          }
          frame Enabled {
          }
        }
        n172 = control-ref of="CH191/FD5 XYZ"() -> (w406:refnum<vi>)
        n173 = control-ref of="CH197/FD4 XYZ"() -> (w404:refnum<vi>)
        n174 = control-ref of="CH1/FD1 XYZ"() -> (w407:refnum<vi>)
        n175 = control-ref of="CH8/FD2 XYZ"() -> (w405:refnum<vi>)
        n176 = Build Array "Build Array"(w407, w406, w405, w404) -> (w410:refnum<vi>[])
        n177 = shared-variable ".\\Component Tray.lvclass\\Camera"() -> (w398:dbl[])  [unwired: 1 in, 1 out]
        n178 = Search 1D Array(1D array=w396, element=TRUE) -> (index of element=w403:i32)  [unwired: 1 in]
        n179 = Index Array "Index Array"(array=w410, index=w403) -> (element=w409:refnum<vi>)
        n180 = Reshape Array(w398, 3 ("dimension size")) -> (w397:dbl[])
        n181 = Add(x=w388, y=w397) -> (x+y=w395:dbl[])
        n182 = Multiply(x=w403, y=3) -> (x*y=w394:i32)
        n183 = property class="Arr (strict)"(reference=w409, error in=w383, "Value"=w395) -> (error out=w390:errorcluster)  [unwired: 1 out]
        n184 = property on="Manual Mode On" class="Bool (strict)"() -> ("Value"=w401:bool)  [unwired: 2 in, 2 out]
        n185 = call "Record Fiducial.vi"("CH index"=w394, "XYZ"=w395, "input cluster"=w385) -> ("All fiducials recorded"=w393:bool, "output cluster"=w392:T7)  [unwired: 7 in]
        "All fiducials recorded" <- w393
        n186 = case shown="True" w393 {
          tunnel: w401 -> [w441 w455]
          tunnel: w392 -> [w440 w454]
          tunnel: w390 -> [w438 w450]
          tunnel: [w437 w449] -> w389
          frame False {
            n187 = Unbundle By Name(w440) -> ("4 fiducials?"=w439:bool)
            n188 = case shown="False" w439 {
              selector: w439 -> [_ w448]
              tunnel: w441 -> [w443 _]
              tunnel: w438 -> [w442 w447]
              tunnel: [w442 w446] -> w437
              frame False {
                n189 = case shown="False" w443 {
                  selector: w443 -> [_ w445]
                  frame False {
                    n190 = property on="Go to CH8/FD2" class="Bool (strict)"("Val(Sgnl)"=TRUE ("Value (Signaling)")) -> ()  [unwired: 2 in, 2 out]
                  }
                  frame True {
                    n191 = property on="Enter Manual Mode" class="Bool (strict)"("Val(Sgnl)"=w445) -> ()  [unwired: 2 in, 2 out]
                  }
                }
              }
              frame True {
                n192 = property on="Predict fiducials" class="Bool (strict)"(error in=w447, "Val(Sgnl)"=w448) -> (error out=w446:errorcluster)  [unwired: 1 in, 1 out]
              }
            }
          }
          frame True {
            n193 = Unbundle By Name(w454) -> ("Sensor ID Location"=→"Sensor ID Location":dbl[], "CH1 Location"=→"CH1 XYZ":dbl[], "XYZTheta"=→"XYZTheta":dbl[])
            n194 = case shown="True" w455 {
              selector: w455 -> [_ w461]
              tunnel: w450 -> [w457 w460]
              tunnel: [w456 w459] -> w449
              frame False {
                n195 = property on="Go to CH1" class="Bool (strict)"(error in=w457, "Val(Sgnl)"=TRUE ("Value (Signaling)")) -> (error out=w456:errorcluster)  [unwired: 1 in, 1 out]
              }
              frame True {
                n196 = property on="Enter Manual Mode" class="Bool (strict)"(error in=w460, "Val(Sgnl)"=w461) -> (error out=w459:errorcluster)  [unwired: 1 in, 1 out]
              }
            }
          }
        }
      }
      event "Predict fiducials": Value Change {
        n197 = event-data() -> ()  [unwired: 1 in, 6 out]
        n198 = property on="Predict fiducials" class="Bool (strict)"("Value"=FALSE ("Predict fiducials")) -> ()  [unwired: 2 in, 2 out]
        n199 = call "Predict Fiducials.vi"("input cluster"=w465) -> ("output cluster"=w464:T7)  [unwired: 10 in]
        n200 = property on="Manual Mode On" class="Bool (strict)"() -> ("Value"=w467:bool)  [unwired: 2 in, 2 out]
        n201 = Unbundle By Name(w464) -> ("New Fiducials"=w466:dbl[], "Past Fiducials"=→"predicted fiducials":dbl[][])
        n202 = case shown="False" w467 {
          selector: w467 -> [_ w486]
          tunnel: w466 -> [w470 _]
          frame False {
            n203 = Search 1D Array(1D array=w470, element=0.0) -> (index of element=w474:i32)  [unwired: 1 in]
            n204 = Divide(x=w474, y=3) -> (x/y=w472:dbl)
            n205 = case shown="1" w472 {
              tunnel: TRUE ("Value (Signaling)") -> [w476 w477 w484 w485]
              tunnel: w470 -> [_ w480 _ _]
              frame 0, Default {
                n206 = property on="Go to CH1/FD1" class="Bool (strict)"("Val(Sgnl)"=w476) -> ()  [unwired: 2 in, 2 out]
              }
              frame 1 {
                n207 = Index Array(array=w480, index=6) -> (element=w481:dbl)
                n208 = Not Equal To 0?(x=w481) -> (x != 0?=w478:bool)
                n209 = case shown="True" w478 {
                  tunnel: w477 -> [w482 w483]
                  frame False {
                    n210 = property on="Go to CH8/FD2" class="Bool (strict)"("Val(Sgnl)"=w482) -> ()  [unwired: 2 in, 2 out]
                  }
                  frame True {
                    n211 = property on="Go to CH191/FD5" class="Bool (strict)"("Val(Sgnl)"=w483) -> ()  [unwired: 2 in, 2 out]
                  }
                }
              }
              frame 2 {
                n212 = property on="Go to CH8/FD2" class="Bool (strict)"("Val(Sgnl)"=w484) -> ()  [unwired: 2 in, 2 out]
              }
              frame 3 {
                n213 = property on="Go to CH197/FD4" class="Bool (strict)"("Val(Sgnl)"=w485) -> ()  [unwired: 2 in, 2 out]
              }
            }
          }
          frame True {
            n214 = property on="Enter Manual Mode" class="Bool (strict)"("Val(Sgnl)"=w486) -> ()  [unwired: 2 in, 2 out]
          }
        }
      }
      event "Joystick": Value Change {
        n215 = event-data() -> ()  [unwired: 1 in, 6 out]
        n216 = call "Joystick.vi"("error in (no error)"=w488, "Joystick"="Joystick", "Gantry In"=w491) -> ("error out"=w487:errorcluster, "Gantry Out"=w489:refnum<k24>)  [unwired: 7 in]
      }
      event "Go to Center": Value Change {
        n217 = event-data() -> ()  [unwired: 1 in, 6 out]
        n218 = disable-structure shown="Enabled" {
          disable-tunnel: w499 -> [w503 w518]
          disable-tunnel: [w502 w515] -> w498
          disable-tunnel: w495 -> [_ w516]
          disable-tunnel: [_ w514] -> w494
          frame Disabled {
            n219 = control-ref of="Joystick"() -> (w504:refnum<vi>)
            n220 = property class="Bool (strict)"(reference=w504) -> (reference out=w505:refnum<vi>, "Value"=w506:bool)  [unwired: 1 in, 1 out]
            n221 = case shown="True" w506 {
              selector: w506 -> [_ w513]
              tunnel: w503 -> [w507 w510]
              tunnel: [w507 w509] -> w502
              tunnel: w505 -> [_ w512]
              frame False {
              }
              frame True {
                n222 = Not(x=w513) -> (.not. x?=w508:bool)
                n223 = call "Joystick.vi"("Joystick"=w508, "Gantry In"=w510) -> ("error out"=w511:errorcluster, "Gantry Out"=w509:refnum<k24>)  [unwired: 8 in]
                n224 = property class="Bool (strict)"(reference=w512, error in=w511, "Value"=w508) -> ()  [unwired: 2 out]
              }
            }
          }
          frame Enabled {
            n225 = call "Joystick.vi"("error in (no error)"=w516, "Joystick"=FALSE, "Gantry In"=w518) -> ("error out"=w514:errorcluster, "Gantry Out"=w515:refnum<k24>)  [unwired: 7 in]
          }
        }
        n226 = Unbundle By Name(w500) -> ("XYZTheta"=w501:dbl[])
        n227 = flat-sequence {
          tunnel: w501 -> [w524]
          tunnel: w498 -> [w523]
          tunnel: [w522] -> w496
          tunnel: [w529] -> w497
          tunnel: w496 -> [w529]
          tunnel: w494 -> [w527]
          tunnel: [w525] -> w493
          frame #0 {
            w521 = T8."Disabled and Grayed Out" ("Disabled")
            n228 = call "ClearXYZTheta Go.vi"("Speed"=300.0, "XYZTheta In"=w524, "Gantry In"=w523) -> ("Gantry Out"=w522:refnum<k24>)  [unwired: 6 in, 2 out]
            n229 = property on="Record CH191/FD5" class="Bool (strict)"("DisabledEnum"=w521) -> ()  [unwired: 2 in, 2 out]
            n230 = property on="Go to CH1/FD1" class="Bool (strict)"("DisabledEnum"=w521) -> ()  [unwired: 2 in, 2 out]
            n231 = property on="Go to CH191/FD5" class="Bool (strict)"("DisabledEnum"=w521) -> ()  [unwired: 2 in, 2 out]
            n232 = property on="Go to CH1" class="Bool (strict)"("DisabledEnum"=w521) -> ()  [unwired: 2 in, 2 out]
            n233 = property on="Record CH8/FD2" class="Bool (strict)"("DisabledEnum"=w521) -> ()  [unwired: 2 in, 2 out]
            n234 = property on="Stop Program" class="Bool"("DisabledEnum"=w521) -> ()  [unwired: 2 in, 2 out]
            n235 = property on="Go to CH197/FD4" class="Bool (strict)"("DisabledEnum"=w521) -> ()  [unwired: 2 in, 2 out]
            n236 = property on="Go to CH8/FD2" class="Bool (strict)"("DisabledEnum"=w521) -> ()  [unwired: 2 in, 2 out]
            n237 = property on="Go to Sensor ID" class="Bool (strict)"("DisabledEnum"=w521) -> ()  [unwired: 2 in, 2 out]
            n238 = property on="Record CH1/FD1" class="Bool (strict)"("DisabledEnum"=w521) -> ()  [unwired: 2 in, 2 out]
            n239 = property on="Go to Center" class="Bool"("DisabledEnum"=w521) -> ()  [unwired: 2 in, 2 out]
            n240 = property on="Record CH197/FD4" class="Bool (strict)"("DisabledEnum"=w521) -> ()  [unwired: 2 in, 2 out]
            n241 = shared-variable ".\\Component Tray.lvclass\\Instructions"("Moving to component center. Wait for movement to stop." ("Value (Signaling)")) -> ()  [unwired: 1 in, 1 out]
          }
          frame #1 {
            n242 = property on="Manual Mode On" class="Bool (strict)"(error in=w527) -> (error out=w526:errorcluster, "Value"=w528:bool)  [unwired: 1 in, 1 out]
            n243 = case shown="False" w528 {
              selector: w528 -> [_ w533]
              tunnel: w526 -> [w530 w532]
              tunnel: [w530 w531] -> w525
              frame False {
              }
              frame True {
                n244 = property on="Enter Manual Mode" class="Bool (strict)"(error in=w532, "Val(Sgnl)"=w533) -> (error out=w531:errorcluster)  [unwired: 1 in, 1 out]
              }
            }
          }
        }
      }
      event "Go to CH1": Value Change {
        n245 = event-data() -> ()  [unwired: 1 in, 6 out]
        n246 = property on="Go to CH1" class="Bool (strict)"(error in=w538, "Value"=FALSE ("Go to CH1")) -> (error out=w539:errorcluster)  [unwired: 1 in, 1 out]
        n247 = disable-structure shown="Enabled" {
          disable-tunnel: w548 -> [w550 w565]
          disable-tunnel: [w549 w564] -> w547
          disable-tunnel: w539 -> [_ w562]
          disable-tunnel: [_ w561] -> w537
          frame Disabled {
            n248 = control-ref of="Joystick"() -> (w551:refnum<vi>)
            n249 = property class="Bool (strict)"(reference=w551) -> (reference out=w552:refnum<vi>, "Value"=w553:bool)  [unwired: 1 in, 1 out]
            n250 = case shown="True" w553 {
              selector: w553 -> [_ w560]
              tunnel: w550 -> [w554 w557]
              tunnel: [w554 w556] -> w549
              tunnel: w552 -> [_ w559]
              frame False {
              }
              frame True {
                n251 = Not(x=w560) -> (.not. x?=w555:bool)
                n252 = call "Joystick.vi"("Joystick"=w555, "Gantry In"=w557) -> ("error out"=w558:errorcluster, "Gantry Out"=w556:refnum<k24>)  [unwired: 8 in]
                n253 = property class="Bool (strict)"(reference=w559, error in=w558, "Value"=w555) -> ()  [unwired: 2 out]
              }
            }
          }
          frame Enabled {
            n254 = call "Joystick.vi"("error in (no error)"=w562, "Joystick"=FALSE, "Gantry In"=w565) -> ("error out"=w561:errorcluster, "Gantry Out"=w564:refnum<k24>)  [unwired: 7 in]
          }
        }
        n255 = flat-sequence {
          tunnel: w547 -> [w577]
          tunnel: [w576] -> w544
          tunnel: w542 -> [w574]
          tunnel: [w566] -> w541
          tunnel: w537 -> [w571]
          tunnel: [w570] -> w534
          tunnel: w544 -> [w603]
          tunnel: [w603] -> w543
          tunnel: w541 -> [w601]
          tunnel: [w600] -> w540
          tunnel: [w599] -> w535
          tunnel: w534 -> [w599]
          tunnel: [w610] -> w546
          tunnel: w543 -> [w610]
          tunnel: w540 -> [w608]
          tunnel: [w607] -> w536
          tunnel: w535 -> [w606]
          frame #0 {
            w575 = T8."Disabled and Grayed Out" ("Disabled")
            n256 = Unbundle By Name(w574) -> ("CH1 check"=w569:T4, "CH1 Location"=w572:dbl[], "Protomodule?"=w570:bool)
            n257 = property on="Record CH191/FD5" class="Bool (strict)"("DisabledEnum"=w575) -> ()  [unwired: 2 in, 2 out]
            n258 = property on="Stop Program" class="Bool"("DisabledEnum"=w575) -> ()  [unwired: 2 in, 2 out]
            n259 = property on="Go to CH1/FD1" class="Bool (strict)"("DisabledEnum"=w575) -> ()  [unwired: 2 in, 2 out]
            n260 = property on="Go to CH1" class="Bool (strict)"("DisabledEnum"=w575) -> ()  [unwired: 2 in, 2 out]
            n261 = property on="Record CH1/FD1" class="Bool (strict)"("DisabledEnum"=w575) -> ()  [unwired: 2 in, 2 out]
            n262 = property on="Go to Center" class="Bool"("DisabledEnum"=w575) -> ()  [unwired: 2 in, 2 out]
            n263 = property on="Go to CH191/FD5" class="Bool (strict)"("DisabledEnum"=w575) -> ()  [unwired: 2 in, 2 out]
            n264 = property on="Go to Sensor ID" class="Bool (strict)"("DisabledEnum"=w575) -> ()  [unwired: 2 in, 2 out]
            n265 = property on="Go to CH197/FD4" class="Bool (strict)"("DisabledEnum"=w575) -> ()  [unwired: 2 in, 2 out]
            n266 = property on="Record CH197/FD4" class="Bool (strict)"("DisabledEnum"=w575) -> ()  [unwired: 2 in, 2 out]
            n267 = property on="Go to CH8/FD2" class="Bool (strict)"("DisabledEnum"=w575) -> ()  [unwired: 2 in, 2 out]
            n268 = property on="Record CH8/FD2" class="Bool (strict)"("DisabledEnum"=w575) -> ()  [unwired: 2 in, 2 out]
            n269 = shared-variable ".\\Component Tray.lvclass\\Instructions"("Moving to CH1. Wait for movement to stop." ("Value (Signaling)"), error in=w571) -> (error out=w568:errorcluster)
            n270 = disable-structure shown="Enabled" {
              disable-tunnel: w577 -> [w583 w598]
              disable-tunnel: [w582 w594] -> w576
              disable-tunnel: w568 -> [w581 w596]
              disable-tunnel: w572 -> [w579 w592]
              disable-tunnel: [_ w584] -> w567
              frame Disabled {
                n271 = call "ClearXYZTheta Go.vi"("error in (no error)"=w581, "Speed"=300.0, "XYZTheta In"=w579, "Gantry In"=w583) -> ("error out"=w580:errorcluster, "Gantry Out"=w582:refnum<k24>)  [unwired: 5 in, 1 out]
              }
              frame Enabled {
                w585 = FALSE ("Increment?")
                n272 = Delete From Array(array=w592, length=1, index=2) -> (deleted portion=w588:dbl[], array with subset deleted=w589:dbl[])
                n273 = Index Array(array=w588) -> (element=w587:dbl)  [unwired: 1 in]
                n274 = call "XY Go.vi"("Increment?"=w585, "error in (no error)"=w596, "Speed"=100.0, "XY In"=w589, "Gantry In"=w598) -> ("error out"=w593:errorcluster, "Gantry Out"=w595:refnum<k24>)  [unwired: 4 in, 1 out]
                n275 = call "Z Go.vi"("Increment"=w585, "error in (no error)"=w593, "Speed In"=10.0, "Position In"=w587, "Gantry In"=w595) -> ("error out"=w584:errorcluster, "Gantry Out"=w594:refnum<k24>)  [unwired: 3 in, 2 out]
              }
            }
            n276 = shared-variable ".\\Component Tray.lvclass\\Machine Vision"(w569, error in=w567) -> (error out=w566:errorcluster)
          }
          frame #1 {
            n277 = case shown="True" w599 {
              frame False {
              }
              frame True {
                n278 = Wait (ms)(milliseconds to wait=u32 1000) -> ()  [unwired: 1 out]
              }
            }
            n279 = shared-variable ".\\Component Tray.lvclass\\Instructions"("Checking for CH1." ("Instructions"), error in=w601) -> (error out=w600:errorcluster)
          }
          frame #2 {
            n280 = case shown="True" TRUE {
              tunnel: [w613 w627] -> w609
              tunnel: w608 -> [w612 w623]
              tunnel: [w611 w625] -> w607
              tunnel: w606 -> [_ w624]
              frame False {
                n281 = Two Button Dialog(message="Is \"1\" visible on the screen?", 1:"No" ("F button name (\"Cancel\")"), 2:"Yes" ("T button name (\"OK\")")) -> (T button?=w613:bool)
                n282 = case shown="True" w613 {
                  selector: w613 -> [_ w622]
                  tunnel: w612 -> [w618 w620]
                  tunnel: [w617 w621] -> w611
                  frame False {
                    n283 = property on="Enter Manual Mode" class="Bool (strict)"(error in=w618, "Val(Sgnl)"=TRUE ("Value (Signaling)")) -> (error out=w617:errorcluster)  [unwired: 1 in, 1 out]
                  }
                  frame True {
                    n284 = property on="Go to Sensor ID" class="Bool (strict)"(error in=w620, "Val(Sgnl)"=w622) -> (error out=w621:errorcluster)  [unwired: 1 in, 1 out]
                  }
                }
              }
              frame True {
                n285 = disable-structure shown="Enabled" {
                  disable-tunnel: [w631 w633] -> w628
                  disable-tunnel: [w630 w632] -> w626
                  disable-tunnel: w623 -> [w629 _]
                  disable-tunnel: w624 -> [_ w637]
                  disable-tunnel: w623 -> [_ w636]
                  frame Disabled {
                    n286 = shared-variable ".\\Component Tray.lvclass\\Match found?"(error in=w629) -> (w631:bool, error out=w630:errorcluster)
                  }
                  frame Enabled {
                    n287 = local read "Image"() -> (w635:T5)
                    n288 = case shown="False" w637 {
                      tunnel: w635 -> [w641 w645]
                      tunnel: w636 -> [w640 w644]
                      tunnel: [w639 w642] -> w634
                      tunnel: [w638 w643] -> w632
                      frame False {
                        n289 = call "Vision Assistant2"("Image In"=w641, "error in"=w640) -> ("Number of Matches (Pattern Matching 1)"=w639:i32, "error out"=w638:errorcluster)  [unwired: 22 in, 2 out]
                      }
                      frame True {
                        n290 = call "Vision Assistant3"("Image In"=w645, "error in"=w644) -> ("Number of Matches (Pattern Matching 1)"=w642:i32, "error out"=w643:errorcluster)  [unwired: 22 in, 2 out]
                      }
                    }
                    n291 = Greater Than 0?(x=w634) -> (x > 0?=w633:bool)
                  }
                }
                n292 = case shown="False" w628 {
                  selector: w628 -> [_ w677]
                  tunnel: [w650 w677] -> w627
                  tunnel: w626 -> [w648 w673]
                  tunnel: [w646 w674] -> w625
                  frame False {
                    n293 = shared-variable ".\\Component Tray.lvclass\\Instructions"("Answer prompts." ("Instructions"), error in=w648) -> (error out=w647:errorcluster)
                    n294 = Two Button Dialog(message="Warning: CH1 was not detected automatically.\nIs \"1\" visible on the screen?", 1:"No" ("F button name (\"Cancel\")"), 2:"Yes" ("T button name (\"OK\")")) -> (T button?=w651:bool)
                    n295 = case shown="False" w651 {
                      selector: w651 -> [w659 w671]
                      tunnel: [w659 w671] -> w650
                      tunnel: w647 -> [w656 w670]
                      tunnel: [w655 w669] -> w646
                      frame False {
                        n296 = Two Button Dialog(message="FInd fiducials manually with joystick or restart the automated program?", 1:"Automatic" ("F button name (\"Cancel\")"), 2:"Manual" ("T button name (\"OK\")")) -> (T button?=w658:bool)
                        n297 = case shown="True" w658 {
                          tunnel: TRUE ("Value (Signaling)") -> [w665 w668]
                          tunnel: w656 -> [w664 w667]
                          tunnel: [w663 w666] -> w655
                          frame False {
                            n298 = property on="Go to CH1/FD1" class="Bool (strict)"(error in=w664, "Val(Sgnl)"=w665) -> (error out=w663:errorcluster)  [unwired: 1 in, 1 out]
                          }
                          frame True {
                            n299 = property on="Enter Manual Mode" class="Bool (strict)"(error in=w667, "Val(Sgnl)"=w668) -> (error out=w666:errorcluster)  [unwired: 1 in, 1 out]
                          }
                        }
                      }
                      frame True {
                        n300 = property on="Go to Sensor ID" class="Bool (strict)"(error in=w670, "Val(Sgnl)"=w671) -> (error out=w669:errorcluster)  [unwired: 1 in, 1 out]
                      }
                    }
                  }
                  frame True {
                    n301 = shared-variable ".\\Component Tray.lvclass\\Instructions"("CH1 automatically detected." ("Instructions"), error in=w673) -> (error out=w672:errorcluster)
                    n302 = property on="Manual Mode On" class="Bool (strict)"(error in=w672) -> (error out=w675:errorcluster, "Value"=w678:bool)  [unwired: 1 in, 1 out]
                    n303 = case shown="False" w678 {
                      selector: w678 -> [_ w684]
                      tunnel: w675 -> [w680 w683]
                      tunnel: [w679 w682] -> w674
                      frame False {
                        n304 = property on="Go to Sensor ID" class="Bool (strict)"(error in=w680, "Val(Sgnl)"=TRUE ("Go to Sensor ID")) -> (error out=w679:errorcluster)  [unwired: 1 in, 1 out]
                      }
                      frame True {
                        n305 = property on="Enter Manual Mode" class="Bool (strict)"(error in=w683, "Val(Sgnl)"=w684) -> (error out=w682:errorcluster)  [unwired: 1 in, 1 out]
                      }
                    }
                  }
                }
              }
            }
            "CH1 correct?" <- w609
          }
        }
      }
      event "Enter Manual Mode": Value Change {
        w693 = T8."Enabled" ("Disabled")
        n306 = event-data() -> ()  [unwired: 1 in, 6 out]
        n307 = Unbundle By Name(w689) -> ("4 fiducials?"=w688:bool)
        n308 = case shown="True" w688 {
          tunnel: [T8."Disabled and Grayed Out" ("Disabled") T8."Enabled" ("Disabled")] -> w692
          frame False {
          }
          frame True {
          }
        }
        n309 = property on="Enter Manual Mode" class="Bool (strict)"("Value"=FALSE ("Enter Manual Mode")) -> ()  [unwired: 2 in, 2 out]
        n310 = local read "Enter Manual Mode"() -> (w685:bool)
        n311 = property on="Go to CH1" class="Bool (strict)"("DisabledEnum"=w693) -> ()  [unwired: 2 in, 2 out]
        n312 = case shown="True" w685 {
          selector: w685 -> [_ w694]
          frame False {
          }
          frame True {
            "Manual Mode On" <- w694
          }
        }
        n313 = shared-variable ".\\Component Tray.lvclass\\Instructions"("Now in manual mode." ("Value (Signaling)")) -> ()  [unwired: 1 in, 1 out]
        n314 = property on="Go to Sensor ID" class="Bool (strict)"("DisabledEnum"=w693) -> ()  [unwired: 2 in, 2 out]
        n315 = property on="Record CH1/FD1" class="Bool (strict)"("DisabledEnum"=w693) -> ()  [unwired: 2 in, 2 out]
        n316 = property on="Go to CH8/FD2" class="Bool (strict)"("DisabledEnum"=w693) -> ()  [unwired: 2 in, 2 out]
        n317 = property on="Go to Center" class="Bool"("DisabledEnum"=w693) -> ()  [unwired: 2 in, 2 out]
        n318 = property on="Record CH8/FD2" class="Bool (strict)"("DisabledEnum"=w693) -> ()  [unwired: 2 in, 2 out]
        n319 = property on="Go to CH1/FD1" class="Bool (strict)"("DisabledEnum"=w693) -> ()  [unwired: 2 in, 2 out]
        n320 = property on="Stop Program" class="Bool"("DisabledEnum"=w693) -> ()  [unwired: 2 in, 2 out]
        n321 = property on="Record CH191/FD5" class="Bool (strict)"("DisabledEnum"=w692) -> ()  [unwired: 2 in, 2 out]
        n322 = property on="Go to CH191/FD5" class="Bool (strict)"("DisabledEnum"=w692) -> ()  [unwired: 2 in, 2 out]
        n323 = property on="Record CH197/FD4" class="Bool (strict)"("DisabledEnum"=w692) -> ()  [unwired: 2 in, 2 out]
        n324 = property on="Go to CH197/FD4" class="Bool (strict)"("DisabledEnum"=w692) -> ()  [unwired: 2 in, 2 out]
      }
      event "Go to Sensor ID": Value Change {
        n325 = event-data() -> ()  [unwired: 1 in, 6 out]
        n326 = flat-sequence {
          tunnel: w706 -> [w711]
          tunnel: w709 -> [w712]
          tunnel: w697 -> [w713]
          tunnel: [w713] -> w703
          tunnel: [w712] -> w701
          tunnel: [w711] -> w699
          tunnel: ["Go to Sensor ID"] -> w704
          tunnel: w703 -> [w718]
          tunnel: [w718] -> w702
          tunnel: w701 -> [w717]
          tunnel: [w717] -> w700
          tunnel: w699 -> [w715]
          tunnel: [w714] -> w698
          tunnel: [w724] -> w707
          tunnel: [w720] -> w705
          tunnel: w702 -> [w723]
          tunnel: w700 -> [w725]
          tunnel: w698 -> [w721]
          tunnel: w697 -> [w719]
          tunnel: [w1226] -> w708
          tunnel: w707 -> [w1226]
          frame #0 {
          }
          frame #1 {
            n327 = property on="Go to Sensor ID" class="Bool (strict)"(error in=w715, "Value"=FALSE ("Go to Sensor ID")) -> (error out=w714:errorcluster)  [unwired: 1 in, 1 out]
          }
          frame #2 {
            n328 = Unbundle By Name(w723) -> ("Protomodule?"=w722:bool)
            n329 = case shown="True" w722 {
              tunnel: w723 -> [_ w773]
              tunnel: w725 -> [w727 w750]
              tunnel: [w727 w772] -> w724
              tunnel: w721 -> [w726 w747]
              tunnel: [w726 w738] -> w720
              tunnel: w719 -> [_ w734]
              frame False {
              }
              frame True {
                w758 = T8."Disabled and Grayed Out" ("Disabled")
                n330 = Unbundle By Name(w773) -> ("Sensor ID Location"=w771:dbl[], "XYZTheta"=w770:dbl[], "Position"=w769:i32, "Pos multiplier"=w754:dbl)
                n331 = Unbundle By Name(w734) -> ("Position"=w733:i32)
                n332 = Multiply(x=-0.44 ("r"), y=w754) -> (x*y=w755:dbl)
                n333 = Index Array(array=w770, index=3) -> (element=w760:dbl)
                n334 = local read "CH197/FD4 XYZ"() -> (w753:dbl[])
                n335 = Array Subset(array=w771, length=2) -> (w761:dbl[])  [unwired: 1 in]
                n336 = Add(x=w760, y=1.5707963267948966) -> (x+y=w765:dbl)
                n337 = local write "Machine Vision"(Machine_Vision."sensor edge init" ("Machine Vision")) -> ()
                n338 = Index Array(array=w753, index=2) -> (element=w751:dbl)
                n339 = for {
                  N: 5 -> [_]
                  shift-right: [w1208] -> _
                  shift-left: w761 -> [w1212]
                  shift-right: [w1211] -> _
                  shift-left: w765 -> [w1211]
                  tunnel: [w1208] -> w764 mode=indexing
                  shift-right: [w1207] -> _
                  shift-left: w755 -> [w1207]
                  n340 = in-place {
                    in-place-border: w1211 -> [w1214]
                    in-place-border: [w1214] -> _
                    in-place-border: w1207 -> [w1213]
                    n341 = in-place-array #2(w1212, 0, 1) -> (w1220:dbl, w1219:dbl)
                    n342 = Polar To Re/Im(2:w1214, 3:w1213) -> (0:w1217:dbl, 1:w1218:dbl)
                    n343 = Add(x=w1220, y=w1218) -> (x+y=w1216:dbl)
                    n344 = Add(x=w1219, y=w1217) -> (x+y=w1215:dbl)
                    n345 = in-place-array #2(w1216, w1215) -> (w1208:dbl[])  [unwired: 2 out]
                  }
                }
                n346 = property on="Go to CH1" class="Bool (strict)"("DisabledEnum"=w758) -> ()  [unwired: 2 in, 2 out]
                n347 = property on="Go to CH1/FD1" class="Bool (strict)"("DisabledEnum"=w758) -> ()  [unwired: 2 in, 2 out]
                n348 = property on="Go to CH191/FD5" class="Bool (strict)"("DisabledEnum"=w758) -> ()  [unwired: 2 in, 2 out]
                n349 = property on="Record CH8/FD2" class="Bool (strict)"("DisabledEnum"=w758) -> ()  [unwired: 2 in, 2 out]
                n350 = property on="Go to CH197/FD4" class="Bool (strict)"("DisabledEnum"=w758) -> ()  [unwired: 2 in, 2 out]
                n351 = property on="Go to CH8/FD2" class="Bool (strict)"("DisabledEnum"=w758) -> ()  [unwired: 2 in, 2 out]
                n352 = property on="Record CH1/FD1" class="Bool (strict)"("DisabledEnum"=w758) -> ()  [unwired: 2 in, 2 out]
                n353 = property on="Record CH191/FD5" class="Bool (strict)"("DisabledEnum"=w758) -> ()  [unwired: 2 in, 2 out]
                n354 = property on="Go to Center" class="Bool"("DisabledEnum"=w758) -> ()  [unwired: 2 in, 2 out]
                n355 = property on="Go to Sensor ID" class="Bool (strict)"("DisabledEnum"=w758) -> ()  [unwired: 2 in, 2 out]
                n356 = property on="Record CH197/FD4" class="Bool (strict)"("DisabledEnum"=w758) -> ()  [unwired: 2 in, 2 out]
                n357 = property on="Stop Program" class="Bool"("DisabledEnum"=w758) -> ()  [unwired: 2 in, 2 out]
                n358 = call "Z Go.vi"("error in (no error)"=w747, "Speed In"=5.0, "Position In"=w751, "Gantry In"=w750) -> ("error out"=w746:errorcluster, "Gantry Out"=w749:refnum<k24>)  [unwired: 4 in, 2 out]
                n359 = shared-variable ".\\Component Tray.lvclass\\Instructions"("Now determining sensor ID. This takes several seconds, please wait." ("Value (Signaling)")) -> ()  [unwired: 1 in, 1 out]
                n360 = Build Array (concatenate)(w761, w764) -> (w762:dbl[][])
                n361 = disable-structure shown="Enabled" {
                  disable-tunnel: [w835 w912 w1010 w1119] -> w772
                  disable-tunnel: w769 -> [w834 _ _ _]
                  disable-tunnel: w762 -> [w828 w911 w1009 w1118]
                  disable-tunnel: w749 -> [w827 w910 w1011 w1120]
                  disable-tunnel: w760 -> [w811 _ _ _]
                  disable-tunnel: [w809 _ w997 w1106] -> w759
                  disable-tunnel: [w808 w896 w1000 w1109] -> w732
                  disable-tunnel: [w807 w905 w1008 w1117] -> w742
                  disable-tunnel: w746 -> [w806 w909 w993 w1105]
                  disable-tunnel: w754 -> [_ w904 w1012 w1121]
                  disable-tunnel: [_ w895 w999 w1108] -> w745
                  frame Disabled {
                    n362 = call "Base File Path.vi"() -> ("Paths Out"=w833:T15)  [unwired: 11 in]
                    n363 = Unbundle By Name(w833) -> ("Components Folder"=w832:path)
                    n364 = Build Path(base path=w832, name or relative path=path "temp") -> (appended path=w831:path)
                    n365 = Create Folder(path (use dialog)=w831, error in=w806) -> (created path=w830:path, error out=w813:errorcluster)  [unwired: 1 in, 1 out]
                    n366 = for {
                      shift-right: [w850] -> w835
                      shift-left: w827 -> [w851]
                      shift-right: [w848] -> w814
                      shift-left: w830 -> [w848]
                      tunnel: w828 -> [w847] mode=indexing
                      shift-right: [w845] -> w812
                      shift-left: w813 -> [w846]
                      tunnel: [w844] -> w809 mode=indexing
                      i -> [w849]
                      n367 = flat-sequence {
                        tunnel: w851 -> [w858]
                        tunnel: [w855] -> w843
                        tunnel: w847 -> [w854]
                        tunnel: w846 -> [w853]
                        tunnel: [w852] -> w842
                        tunnel: w843 -> [w869]
                        tunnel: [w869] -> w841
                        tunnel: w849 -> [w865]
                        tunnel: w848 -> [w862]
                        tunnel: [w861] -> w840
                        tunnel: [w859] -> w839
                        tunnel: w842 -> [w859]
                        tunnel: w841 -> [w875]
                        tunnel: w840 -> [w871]
                        tunnel: w839 -> [w874]
                        tunnel: [w875] -> w838
                        tunnel: [w873] -> w837
                        tunnel: [w871] -> w836
                        tunnel: [w877] -> w845
                        tunnel: [w880] -> w850
                        tunnel: w838 -> [w880]
                        tunnel: w837 -> [w878]
                        tunnel: w836 -> [w879]
                        tunnel: [w876] -> w844
                        frame #0 {
                          n368 = call "XY Go.vi"("return immediately"=FALSE, "error in (no error)"=w853, "Speed"=100.0, "XY In"=w854, "Gantry In"=w858) -> ("error out"=w852:errorcluster, "Gantry Out"=w855:refnum<k24>)  [unwired: 4 in, 1 out]
                        }
                        frame #1 {
                          n369 = Wait (ms)(milliseconds to wait=u32 1000) -> ()  [unwired: 1 out]
                          n370 = Number To Decimal String(number=w865) -> (decimal integer string=w867:string)  [unwired: 1 in]
                          n371 = Concatenate Strings("temp" ("string"), w867, ".bmp" ("string")) -> (w868:string)
                          n372 = String To Path(string=w868) -> (path=w866:path)
                          n373 = Build Path(base path=w862, name or relative path=w866) -> (appended path=w861:path)
                        }
                        frame #2 {
                          n374 = local read "Image"() -> (w870:T5)
                          n375 = Wait (ms)(milliseconds to wait=u32 1000) -> ()  [unwired: 1 out]
                          n376 = call-poly "IMAQ Write File 2"("error in (no error)"=w874, "File Path"=w871, "Image"=w870) -> ("error out"=w873:errorcluster)  [unwired: 7 in, 1 out]
                        }
                        frame #3 {
                          n377 = disable-structure shown="Enabled" {
                            disable-tunnel: w879 -> [w887 w893]
                            disable-tunnel: w878 -> [w886 w892]
                            disable-tunnel: [w885 w891] -> w877
                            disable-tunnel: [w883 w894] -> w876
                            frame Disabled {
                              n378 = call <vilib>:"Read BMP File.vi"("error in (no error)"=w886, "path to BMP file"=w887) -> ("error out"=w885:errorcluster, "image data"=w882:T16)  [unwired: 7 in, 1 out]
                              n379 = in-place {
                                n380 = in-place-cluster #3(w882) -> ("Rectangle"=w890:T13)
                                n381 = Divide(x=w890, y=T13 {"left"=2, "top"=2, "right"=2, "bottom"=2}) -> (x/y=w888:T17)
                                n382 = in-place-cluster #3("Rectangle"=w888) -> (w881:T16)
                              }
                              n383 = call <vilib>:"Draw Flattened Pixmap.vi"("image data"=w881, "picture"=picture data[5B]) -> ("new picture"=w883:picture)  [unwired: 7 in]
                            }
                            frame Enabled {
                              n384 = call "Resize Image to a Container 2012 NIVerified.vi"("error in (no error)"=w892, "Path to Image (PNG, JPEG, BMP)"=w893) -> ("error out"=w891:errorcluster, "Resized Image"=w894:picture)  [unwired: 7 in]
                            }
                          }
                        }
                      }
                    }
                    n385 = call "Base File Path.vi"() -> ("Paths Out"=w822:T15)  [unwired: 11 in]
                    n386 = Unbundle By Name(w822) -> ("Components Folder"=w821:path)
                    n387 = call "Get Python Version.vi"("error in (no error)"=w812) -> ("Python Version"=w818:string, "error out"=w817:errorcluster)  [unwired: 9 in]
                    n388 = Build Path(base path=w821, name or relative path=path "SensorID.py") -> (appended path=w820:path)
                    n389 = Path To String(path=w814) -> (string=w815:string)
                    n390 = Open Python Session(python version=w818, 3:w817) -> (session out=w826:refnum<k35>, error out=w824:errorcluster)  [unwired: 1 in]
                    n391 = node(w826, w820, "read_sensor_ID" ("function name"), w824, "read_sensor_ID" ("string"), w815, w834, w811) -> (w825:refnum<k35>, w823:errorcluster, w808:string)  [unwired: 3 in, 2 out]
                    n392 = Close Python Session(session in=w825, error in=w823) -> (11:w807:errorcluster)
                  }
                  frame Disabled {
                    n393 = for {
                      shift-right: [w975] -> w912
                      shift-left: w910 -> [w976]
                      tunnel: w911 -> [w974] mode=indexing
                      shift-right: [w972] -> w906
                      shift-left: w909 -> [w973]
                      tunnel: [w967] -> w908 mode=indexing
                      n394 = flat-sequence {
                        tunnel: w976 -> [w983]
                        tunnel: [w980] -> w969
                        tunnel: w974 -> [w979]
                        tunnel: w973 -> [w978]
                        tunnel: [w977] -> w968
                        tunnel: w969 -> [w986]
                        tunnel: w968 -> [w985]
                        tunnel: [w986] -> w971
                        tunnel: [w985] -> w970
                        tunnel: [w988] -> w972
                        tunnel: [w989] -> w975
                        tunnel: w971 -> [w989]
                        tunnel: w970 -> [w988]
                        tunnel: [w987] -> w967
                        frame #0 {
                          n395 = call "XY Go.vi"("return immediately"=FALSE, "error in (no error)"=w978, "Speed"=100.0, "XY In"=w979, "Gantry In"=w983) -> ("error out"=w977:errorcluster, "Gantry Out"=w980:refnum<k24>)  [unwired: 4 in, 1 out]
                        }
                        frame #1 {
                          n396 = Wait (ms)(milliseconds to wait=u32 1000) -> ()  [unwired: 1 out]
                        }
                        frame #2 {
                          n397 = local read "Image"() -> (w987:T5)
                        }
                      }
                    }
                    n398 = for {
                      tunnel: w908 -> [w926] mode=indexing
                      tunnel: T5 refnum ("Template Image") -> [w925]
                      shift-right: [w923] -> w905
                      shift-left: w906 -> [w924]
                      tunnel: w904 -> [w916]
                      tunnel: [w914] -> w897 mode=indexing
                      tunnel: [w913] -> w895 mode=indexing
                      n399 = call "IMAQ Match Pattern 4"("Image"=w926, "Algorithm"="Algorithm", "Template Image"=w925, "ROI Descriptor"="ROI Descriptor", "Parameters"="Parameters", "error in (no error)"=w924, "Advanced Options"="Advanced Options") -> ("Matches (real-world)"=w915:T18, "Number of Matches"=w918:i32, "error out"=w923:errorcluster)  [unwired: 4 in, 2 out]
                      n400 = Greater Than 0?(x=w918) -> (x > 0?=w917:bool)
                      n401 = case shown="False" w917 {
                        tunnel: w916 -> [w930 _]
                        tunnel: [w928 0 ("index")] -> w913
                        tunnel: w915 -> [w927 _]
                        frame False {
                          n402 = for {
                            tunnel: w930 -> [w939]
                            tunnel: [w938] -> w929 mode=indexing
                            tunnel: w927 -> [w933] mode=indexing
                            n403 = Unbundle By Name(w933) -> ("Position"=w932:cluster{"x":sgl, "y":sgl})
                            n404 = Cluster To Array(cluster=w932) -> (array=w931:sgl[])
                            n405 = Index Array(array=w931, index #1=0 ("index"), index #2=1 ("index")) -> (element #2=w940:sgl)  [unwired: 1 out]
                            n406 = Multiply(x=w940, y=w939) -> (x*y=w936:dbl)
                            n407 = Absolute Value(x=w936) -> (abs(x)=w935:dbl)
                            n408 = Greater?(x=w935, y=0.25) -> (0:w934:bool)
                            n409 = case shown="False" w934 {
                              tunnel: w936 -> [w944 _]
                              tunnel: [w943 0 ("index")] -> w938
                              frame False {
                                n410 = Greater?(x=w944, y=0.1) -> (0:w946:bool)
                                n411 = case shown="False" w946 {
                                tunnel: w944 -> [w948 _]
                                tunnel: [w947 8 ("index")] -> w943
                                frame False {
                                n412 = Greater?(x=w948, y=0.01) -> (0:w950:bool)
                                n413 = case shown="False" w950 {
                                tunnel: w948 -> [w955 _]
                                tunnel: [w952 4 ("index")] -> w947
                                frame False {
                                n414 = Negate(x=w955) -> (-x=w951:dbl)
                                n415 = Greater?(x=w951, y=0.1) -> (0:w953:bool)
                                n416 = case shown="False" w953 {
                                tunnel: [w956 1 ("index")] -> w952
                                tunnel: w951 -> [w958 _]
                                frame False {
                                n417 = Greater?(x=w958, y=0.01) -> (0:w957:bool)
                                n418 = case shown="True" w957 {
                                tunnel: [0 ("index") 2 ("index")] -> w956
                                frame False {
                                }
                                frame True {
                                }
                                }
                                }
                                frame True {
                                }
                                }
                                }
                                frame True {
                                }
                                }
                                }
                                frame True {
                                }
                                }
                              }
                              frame True {
                              }
                            }
                          }
                          n419 = Add Array Elements(numeric array=w929) -> (sum=w928:i32)
                        }
                        frame True {
                        }
                      }
                      n420 = Number To Decimal String(number=w913) -> (decimal integer string=w914:string)  [unwired: 1 in]
                    }
                    n421 = Index Array(array=w897) -> (element #1=w903:string, element #2=w902:string, element #3=w901:string, element #4=w900:string, element #5=w899:string, element #6=w898:string)  [unwired: 6 in]
                    n422 = Concatenate Strings(w903, w902, w901, w900, w899, w898) -> (w896:string)
                  }
                  frame Disabled {
                    n423 = call "IMAQ Learn Pattern 6"("Image"=T5 refnum, "error in (no error)"=w993) -> ("Template Image Out"=w990:T5, "error out"=w992:errorcluster)  [unwired: 11 in, 1 out]
                    n424 = property on="new picture" class="Pict"(error in=w992, "ZoomFactor"=sgl 0.1 ("Zoom Factor")) -> (error out=w996:errorcluster)  [unwired: 1 in, 1 out]
                    n425 = property on="Machine Vision" class="Enum (strict)"(error in=w996, "Val(Sgnl)"=Machine_Vision."sensor ID" ("Value (Signaling)")) -> (error out=w994:errorcluster)  [unwired: 1 in, 1 out]
                    n426 = for {
                      tunnel: w1012 -> [w1024]
                      shift-right: [w1021] -> w1010
                      shift-left: w1011 -> [w1023]
                      shift-right: [w1015] -> w1008
                      shift-left: w994 -> [w1022]
                      tunnel: w1009 -> [w1020] mode=indexing
                      tunnel: [w1019] -> w1007 mode=indexing
                      tunnel: [w1018] -> w999 mode=indexing
                      tunnel: [w1016] -> w997 mode=indexing
                      tunnel: w990 -> [w1013]
                      n427 = flat-sequence {
                        tunnel: w1023 -> [w1029]
                        tunnel: [w1028] -> w1021
                        tunnel: w1022 -> [w1027]
                        tunnel: w1020 -> [w1026]
                        tunnel: [w1025] -> w1014
                        tunnel: [w1031] -> w1017
                        tunnel: w1014 -> [w1031]
                        tunnel: w1024 -> [w1055]
                        tunnel: [w1050] -> w1018
                        tunnel: w1013 -> [w1040]
                        tunnel: [w1041] -> w1015
                        tunnel: [w1047] -> w1016
                        tunnel: w1017 -> [w1045]
                        frame #0 {
                          n428 = call "XY Go.vi"("error in (no error)"=w1027, "Speed"=100.0, "XY In"=w1026, "Gantry In"=w1029) -> ("error out"=w1025:errorcluster, "Gantry Out"=w1028:refnum<k24>)  [unwired: 5 in, 1 out]
                        }
                        frame #1 {
                          n429 = Wait (ms)(milliseconds to wait=u32 1000) -> ()  [unwired: 1 out]
                        }
                        frame #2 {
                          w1039 = i32[] [800, 300, 1700, 1500] ("Optional Rectangle")
                          n430 = local read "Image"() -> (w1048:T5)
                          n431 = Build Array (concatenate)(w1039, i32[] [] ("array")) -> (w1037:i32[])
                          n432 = call <vilib>:"IMAQdx Snap2.vi"("error in"=w1045, "Image In"=w1048) -> ("error out"=w1044:errorcluster, "Image Out"=w1043:T5)  [unwired: 7 in, 1 out]
                          n433 = Array To Cluster(array=w1037) -> (cluster=w1036:T19)
                          n434 = call "IMAQ ImageToArray"("error in (no error)"=w1044, "Optional Rectangle"=w1039, "Image"=w1048) -> ("error out"=w1042:errorcluster, "Image Pixels (U8)"=w1046:u8[][])  [unwired: 1 in, 3 out]
                          n435 = disable-structure shown="Enabled" {
                            disable-tunnel: [w1058 w1061] -> w1047
                            disable-tunnel: w1046 -> [w1057 w1062]
                            frame Disabled {
                              n436 = call <vilib>:"Flatten Pixmap.vi"("8-bit pixmap"=w1057) -> ("image data"=w1059:T16)  [unwired: 10 in]
                              n437 = call <vilib>:"Draw Flattened Pixmap.vi"("image data"=w1059, "picture"=picture data[5B]) -> ("new picture"=w1058:picture)  [unwired: 7 in]
                            }
                            frame Enabled {
                              n438 = call-poly <vilib>:"Draw Unflattened Pixmap.vi"("picture"=picture data[5B], "data"=w1062) -> ("new picture"=w1061:picture)  [unwired: 7 in]
                            }
                          }
                          n439 = call "IMAQ Find Pattern 4"("Image"=w1043, "Template"=w1040, "Search Rect"=w1036, "error in"=w1042, "Settings"=T14 {"Algorithm"=2, "Number of Matches Requested"=3, "Minimum Match Score"=800.0, "SubPixel Accuracy"=TRUE, "Rotation Angle Ranges"=[{"Start"=0.0, "End"=180.0}], "Show Search Area"=TRUE, "Show Result"=TRUE}) -> ("Number of Matches"=w1034:i32, "Matches (real-world)"=w1033:T18, "error out"=w1041:errorcluster)  [unwired: 4 in, 4 out]
                          n440 = Equal To 0?(x=w1034) -> (x = 0?=w1054:bool)
                          n441 = Initialize Array(FALSE, 4 ("dimension size")) -> (w1053:bool[])
                          n442 = case shown="False" w1054 {
                            tunnel: w1055 -> [w1066 _]
                            tunnel: w1053 -> [w1065 w1101]
                            tunnel: [w1064 w1101] -> w1049
                            tunnel: w1033 -> [w1063 _]
                            frame False {
                              n443 = for {
                                tunnel: w1066 -> [w1076]
                                shift-right: [w1070] -> w1064
                                shift-left: w1065 -> [w1071]
                                tunnel: w1063 -> [w1069] mode=indexing
                                n444 = Unbundle By Name(w1069) -> ("Position"=w1068:cluster{"x":sgl, "y":sgl})
                                n445 = Cluster To Array(cluster=w1068) -> (array=w1067:sgl[])
                                n446 = Index Array(array=w1067, index #1=0 ("index"), index #2=1 ("index")) -> (element #2=w1077:sgl)  [unwired: 1 out]
                                n447 = Multiply(x=w1077, y=w1076) -> (x*y=w1074:dbl)
                                n448 = Absolute Value(x=w1074) -> (abs(x)=w1073:dbl)
                                n449 = Greater?(x=w1073, y=0.25) -> (0:w1072:bool)
                                n450 = case shown="False" w1072 {
                                tunnel: w1074 -> [w1084 _]
                                tunnel: w1071 -> [w1083 w1100]
                                tunnel: [w1080 w1100] -> w1070
                                frame False {
                                n451 = Greater?(x=w1084, y=0.1) -> (0:w1086:bool)
                                n452 = case shown="False" w1086 {
                                tunnel: w1084 -> [w1088 _]
                                tunnel: [w1087 3 ("index")] -> w1081
                                frame False {
                                n453 = Greater?(x=w1088, y=0.01) -> (0:w1090:bool)
                                n454 = case shown="False" w1090 {
                                tunnel: w1088 -> [w1095 _]
                                tunnel: [w1092 2 ("index")] -> w1087
                                frame False {
                                n455 = Negate(x=w1095) -> (-x=w1091:dbl)
                                n456 = Greater?(x=w1091, y=0.1) -> (0:w1093:bool)
                                n457 = case shown="True" w1093 {
                                tunnel: [1 ("index") 0 ("index")] -> w1092
                                frame False {
                                }
                                frame True {
                                }
                                }
                                }
                                frame True {
                                }
                                }
                                }
                                frame True {
                                }
                                }
                                n458 = Replace Array Subset(array=w1083, new element=TRUE ("new element/subarray"), index=w1081) -> (w1080:bool[])
                                }
                                frame True {
                                }
                                }
                              }
                            }
                            frame True {
                            }
                          }
                          n459 = Boolean Array To Number(Boolean array=w1049) -> (number=w1050:u32)
                        }
                      }
                      n460 = Number To Decimal String(number=w1018) -> (decimal integer string=w1019:string)  [unwired: 1 in]
                    }
                    n461 = Index Array(array=w1007) -> (element #1=w1006:string, element #2=w1005:string, element #3=w1004:string, element #4=w1003:string, element #5=w1002:string, element #6=w1001:string)  [unwired: 6 in]
                    n462 = Concatenate Strings(w1006, w1005, w1004, w1003, w1002, w1001) -> (w1000:string)
                  }
                  frame Enabled {
                    n463 = property on="new picture" class="Pict"(error in=w1105, "ZoomFactor"=sgl 0.1 ("Zoom Factor")) -> (error out=w1104:errorcluster)  [unwired: 1 in, 1 out]
                    n464 = property on="Machine Vision" class="Enum (strict)"(error in=w1104, "Val(Sgnl)"=Machine_Vision."sensor ID" ("Value (Signaling)")) -> (error out=w1103:errorcluster)  [unwired: 1 in, 1 out]
                    n465 = for {
                      tunnel: w1121 -> [w1132]
                      shift-right: [w1129] -> w1119
                      shift-left: w1120 -> [w1131]
                      shift-right: [w1122] -> w1117
                      shift-left: w1103 -> [w1130]
                      tunnel: w1118 -> [w1128] mode=indexing
                      tunnel: [w1127] -> w1116 mode=indexing
                      tunnel: [w1126] -> w1108 mode=indexing
                      tunnel: [w1123] -> w1106 mode=indexing
                      n466 = flat-sequence {
                        tunnel: [w1138] -> w1124
                        tunnel: w1131 -> [w1136]
                        tunnel: [w1135] -> w1129
                        tunnel: w1130 -> [w1134]
                        tunnel: w1128 -> [w1133]
                        tunnel: [w1139] -> w1125
                        tunnel: w1124 -> [w1139]
                        tunnel: w1125 -> [w1145]
                        tunnel: [w1143] -> w1123
                        tunnel: [w1148] -> w1122
                        tunnel: [w1152] -> w1126
                        tunnel: w1132 -> [w1156]
                        frame #0 {
                          n467 = call "XY Go.vi"("error in (no error)"=w1134, "Speed"=100.0, "XY In"=w1133, "Gantry In"=w1136) -> ("error out"=w1138:errorcluster, "Gantry Out"=w1135:refnum<k24>)  [unwired: 5 in, 1 out]
                        }
                        frame #1 {
                          n468 = Wait (ms)(milliseconds to wait=u32 1000) -> ()  [unwired: 1 out]
                        }
                        frame #2 {
                          n469 = local read "Image"() -> (w1149:T5)
                          n470 = call "IMAQ ImageToArray"("error in (no error)"=w1145, "Optional Rectangle"=i32[] [800, 300, 1700, 1500], "Image"=w1149) -> ("error out"=w1150:errorcluster, "Image Pixels (U8)"=w1142:u8[][])  [unwired: 1 in, 3 out]
                          n471 = disable-structure shown="Enabled" {
                            disable-tunnel: w1149 -> [w1163 _]
                            disable-tunnel: [w1162 w1169] -> w1148
                            disable-tunnel: w1150 -> [w1161 w1169]
                            disable-tunnel: [w1159 w1168] -> w1147
                            disable-tunnel: [w1157 w1167] -> w1146
                            frame Enabled {
                              n472 = call "Vision Assistant"("Image In"=w1163, "error in"=w1161) -> ("Number of Matches (Pattern Matching 1)"=w1158:i32, "Calibrated Matches (Pattern Matching 1)"=w1160:T18, "error out"=w1162:errorcluster)  [unwired: 22 in, 1 out]
                              n473 = for {
                                tunnel: w1160 -> [w1166] mode=indexing
                                tunnel: [w1164] -> w1159 mode=indexing
                                n474 = Unbundle By Name(w1166) -> ("Position"=w1165:cluster{"x":sgl, "y":sgl})
                                n475 = Cluster To Array(cluster=w1165) -> (array=w1164:sgl[])
                              }
                              n476 = Equal To 0?(x=w1158) -> (x = 0?=w1157:bool)
                            }
                            frame Disabled {
                              n477 = local read "All Matches XY"() -> (w1168:sgl[][])
                              n478 = Empty Array?(array=w1168) -> (empty?=w1167:bool)
                            }
                          }
                          n479 = call-poly <vilib>:"Draw Unflattened Pixmap.vi"("picture"=picture data[5B], "data"=w1142) -> ("new picture"=w1143:picture)  [unwired: 7 in]
                          n480 = Initialize Array(FALSE, 4 ("dimension size")) -> (w1155:bool[])
                          n481 = case shown="False" w1146 {
                            tunnel: w1156 -> [w1173 _]
                            tunnel: w1147 -> [w1172 _]
                            tunnel: w1155 -> [w1171 w1206]
                            tunnel: [w1170 w1206] -> w1151
                            frame False {
                              n482 = for {
                                tunnel: w1172 -> [w1184] mode=indexing
                                tunnel: w1173 -> [w1180]
                                shift-right: [w1174] -> w1170
                                shift-left: w1171 -> [w1175]
                                n483 = Index Array(array=w1184, index #1=0 ("index"), index #2=1 ("index")) -> (element #2=w1181:sgl)  [unwired: 1 out]
                                n484 = Multiply(x=w1181, y=w1180) -> (x*y=w1178:dbl)
                                n485 = Absolute Value(x=w1178) -> (abs(x)=w1177:dbl)
                                n486 = Greater?(x=w1177, y=0.25) -> (0:w1176:bool)
                                n487 = case shown="False" w1176 {
                                tunnel: w1178 -> [w1189 _]
                                tunnel: w1175 -> [w1188 w1205]
                                tunnel: [w1185 w1205] -> w1174
                                frame False {
                                n488 = Greater?(x=w1189, y=0.1) -> (0:w1191:bool)
                                n489 = case shown="False" w1191 {
                                tunnel: w1189 -> [w1193 _]
                                tunnel: [w1192 3 ("index")] -> w1186
                                frame False {
                                n490 = Greater?(x=w1193, y=0.01) -> (0:w1195:bool)
                                n491 = case shown="False" w1195 {
                                tunnel: w1193 -> [w1200 _]
                                tunnel: [w1197 2 ("index")] -> w1192
                                frame False {
                                n492 = Negate(x=w1200) -> (-x=w1196:dbl)
                                n493 = Greater?(x=w1196, y=0.1) -> (0:w1198:bool)
                                n494 = case shown="True" w1198 {
                                tunnel: [1 ("index") 0 ("index")] -> w1197
                                frame False {
                                }
                                frame True {
                                }
                                }
                                }
                                frame True {
                                }
                                }
                                }
                                frame True {
                                }
                                }
                                n495 = Replace Array Subset(array=w1188, new element=TRUE ("new element/subarray"), index=w1186) -> (w1185:bool[])
                                }
                                frame True {
                                }
                                }
                              }
                            }
                            frame True {
                            }
                          }
                          n496 = Boolean Array To Number(Boolean array=w1151) -> (number=w1152:u32)
                        }
                      }
                      n497 = Number To Decimal String(number=w1126) -> (decimal integer string=w1127:string)  [unwired: 1 in]
                    }
                    n498 = Index Array(array=w1116) -> (element #1=w1115:string, element #2=w1114:string, element #3=w1113:string, element #4=w1112:string, element #5=w1111:string, element #6=w1110:string)  [unwired: 6 in]
                    n499 = Concatenate Strings(w1115, w1114, w1113, w1112, w1111, w1110) -> (w1109:string)
                  }
                }
                "Sensor ID" <- w732
                "Sensor ID" <- w759
                "Sensor ID digits" <- w745
                n500 = Decrement(x=w733) -> (x-1=w731:i32)
                n501 = call-dynamic "Read Top Layer ID.vi"("error in (no error)"=w742, "Database Entry in"="Database Entry in") -> ("error out"=w739:errorcluster, "Top Layer IDs"=w735:string[], "Database Entry out"=w737:refnum<class "Database Entry.lvclass">)  [unwired: 7 in]
                n502 = Index Array(array=w735, index=w731) -> (element=w730:string)
                n503 = Search/Split String(string=w730, search string/char (-)="_") -> (substring before match=w728:string)  [unwired: 1 in, 2 out]
                n504 = Equal?(x=w732, y=w728) -> (x = y?=w741:bool)
                n505 = case shown="False" w741 {
                  selector: w741 -> [_ w805]
                  tunnel: [w802 w805] -> w740
                  tunnel: w728 -> [w797 _]
                  frame False {
                    n506 = Empty String/Path?(string/path=w797) -> (empty?=w798:bool)
                    n507 = Select(t="000000", s=w798, f=w797) -> (s? t:f=w795:string)
                    n508 = Concatenate Strings("Warning: Sensor ID did not automatically match with the DB entry.\nDo the thumbnails show ID " ("message"), w795, "?" ("string")) -> (w803:string)
                    n509 = Two Button Dialog(message=w803, 1:"No" ("F button name (\"Cancel\")"), 2:"Yes" ("T button name (\"OK\")")) -> (T button?=w802:bool)
                  }
                  frame True {
                  }
                }
                "Sensor ID match DB?" <- w740
                n510 = case shown="False" w740 {
                  tunnel: w739 -> [w786 w794]
                  tunnel: [w784 w794] -> w738
                  tunnel: w737 -> [w783 w793]
                  tunnel: [w785 w793] -> w736
                  tunnel: w731 -> [w778 _]
                  frame False {
                    n511 = while {
                      tunnel: [w788] -> w775
                      shift-right: [w791] -> w782
                      shift-left: w786 -> [w792]
                      stop <- w787 stop-if-true
                      n512 = call "Prompt User for Input2"("error in (no error)"=w792) -> ("Sensor ID"=w788:string, "error out"=w791:errorcluster)  [unwired: 16 in, 1 out]
                      n513 = String Length(string=w788) -> (length=w790:i32)
                      n514 = Equal?(x=w790, y=6) -> (x = y?=w787:bool)
                    }
                    n515 = Concatenate Strings(w775, "_0" ("string")) -> (w774:string)
                    n516 = call-dynamic "Read New Top Layer ID.vi"("error in (no error)"=w782, "Database Entry in"=w783) -> ("error out"=w781:errorcluster, "Revised Sensor IDs"=w780:string[], "Database Entry out"=w779:refnum<class "Database Entry.lvclass">)  [unwired: 7 in]
                    n517 = Insert Into Array(array=w780, index=w778, new element=w774) -> (w777:string[])
                    n518 = call-dynamic "Write New Top Layer ID.vi"("error in (no error)"=w781, "Revised Sensor IDs"=w777, "Database Entry in"=w779) -> ("error out"=w784:errorcluster, "Database Entry out"=w785:refnum<class "Database Entry.lvclass">)  [unwired: 7 in]
                  }
                  frame True {
                  }
                }
                "Database Entry out" <- w736
              }
            }
          }
          frame #3 {
            n519 = local write "Checking Sensor ID"(FALSE ("Checking Sensor ID")) -> ()
            n520 = Two Button Dialog(message="Ready to Submit?", 1:"No" ("F button name (\"Cancel\")"), 2:"Yes" ("T button name (\"OK\")")) -> (T button?=w1222:bool)
            n521 = case shown="True" w1222 {
              selector: w1222 -> [_ w1228]
              frame False {
                n522 = property on="Enter Manual Mode" class="Bool (strict)"("Val(Sgnl)"=TRUE ("Value (Signaling)")) -> ()  [unwired: 2 in, 2 out]
              }
              frame True {
                n523 = property on="Auto Submit" class="Bool (strict)"("Val(Sgnl)"=w1228) -> ()  [unwired: 2 in, 2 out]
              }
            }
          }
        }
        "Checking Sensor ID" <- w704
      }
    }
    n524 = Equal?(x=w104, y=0) -> (x = y?=w102:bool)
    n525 = case shown="True" w102 {
      tunnel: w101 -> [_ w122]
      tunnel: w100 -> [_ w114]
      frame False {
      }
      frame True {
        w119 = T8."Disabled and Grayed Out" ("Disabled")
        n526 = Unbundle By Name(w114) -> ("Assembly Type"=w113:string, "Tray Number"=w112:string)
        n527 = property on="Go to CH1" class="Bool (strict)"("DisabledEnum"=w119) -> ()  [unwired: 2 in, 2 out]
        n528 = shared-variable ".\\Component Tray.lvclass\\Machine Vision"(T9."Assembly Tray Circle" ("Machine Vision")) -> ()  [unwired: 1 in, 1 out]
        n529 = Format Into String(format string="%d", initial string="Now measuring Position ", w122) -> (resulting string=w118:string)  [unwired: 1 in, 1 out]
        n530 = property on="Stop Program" class="Bool"("DisabledEnum"=w119) -> ()  [unwired: 2 in, 2 out]
        n531 = property on="Record CH197/FD4" class="Bool (strict)"("DisabledEnum"=w119) -> ()  [unwired: 2 in, 2 out]
        n532 = property on="Go to CH8/FD2" class="Bool (strict)"("DisabledEnum"=w119) -> ()  [unwired: 2 in, 2 out]
        n533 = property on="Record CH8/FD2" class="Bool (strict)"("DisabledEnum"=w119) -> ()  [unwired: 2 in, 2 out]
        n534 = property on="Record CH1/FD1" class="Bool (strict)"("DisabledEnum"=w119) -> ()  [unwired: 2 in, 2 out]
        n535 = property on="Go to CH197/FD4" class="Bool (strict)"("DisabledEnum"=w119) -> ()  [unwired: 2 in, 2 out]
        n536 = property on="Go to CH191/FD5" class="Bool (strict)"("DisabledEnum"=w119) -> ()  [unwired: 2 in, 2 out]
        n537 = property on="Go to Center" class="Bool"("DisabledEnum"=w119) -> ()  [unwired: 2 in, 2 out]
        n538 = property on="Go to Sensor ID" class="Bool (strict)"("DisabledEnum"=w119) -> ()  [unwired: 2 in, 2 out]
        n539 = property on="Record CH191/FD5" class="Bool (strict)"("DisabledEnum"=w119) -> ()  [unwired: 2 in, 2 out]
        n540 = property on="Go to CH1/FD1" class="Bool (strict)"("DisabledEnum"=w119) -> ()  [unwired: 2 in, 2 out]
        n541 = shared-variable ".\\Component Tray.lvclass\\Instructions"("Answer prompts then wait for gantry movement." ("Instructions")) -> (error out=w111:errorcluster)  [unwired: 1 in]
        n542 = Concatenate Strings(w118, " on Tray " ("string"), w112, " for " ("string"), w113) -> (→"Tray and Position":string)
        n543 = property on="Go to CH1/FD1" class="Bool (strict)"(error in=w111, "Val(Sgnl)"=TRUE ("Value (Signaling)")) -> ()  [unwired: 1 in, 2 out]
      }
    }
  }
  "Gantry Out" <- w14
